vi "CreateMethod.vi"(0 "ClassWriterNative.lvclass":refnum<class "ClassWriterNative.lvclass">=refnum, 1 "ClassItemRefIn":refnum<vi>, 2 "CreateMethodData":T1={"MethodName"="", "RelativeMethodPath"=path "", "MethodDescription"="", "Scope/Visibility"=enum."Use Parent Folder Scope", "MethodTemplateName"="", "IconOut"=[], "RelativeProjectClassPath"="", "OpenViAfterCreation"=FALSE, "DynamicDispatchVi"=FALSE, "ExtraCreateParameters"=variant, "MustOverride"=FALSE, "MustCallParent"=FALSE, "IconDetails"={"IconSize"=enum."1 c-term high", "ImageRows(32)"=32, "ConnectorPaneHeight"=[]}, "AF-Option"=variant, "TemplatePath"=path ""} {"IconOut" format="%x"}, 5 "error in (no error)":errorcluster) -> (14 "ClassWriterNative.lvclass 2":refnum<class "ClassWriterNative.lvclass">, 15 "ClassItemRefOut":refnum<vi>, 16 "MethodPaths":path[](array[path]), 19 "error out":errorcluster)   [LabVIEW 2020, in "ClassWriterNative.lvclass"]
uses:
  ClassWriterNative.lvclass
  <vilib>/regexp/Match Regular Expression.xnode
  <vilib>/picture/picture.llb/imagedata.ctl
  <resource>/Framework/Providers/Open_GDS/ClassProviders/Common/LvIcon_class/GDSLvIcon_WordCompressionType.ctl
  <resource>/Framework/Providers/Open_GDS/ClassProviders/Common/LvIcon_class/subvis/GDSLvIcon_TextDataType.ctl
  <resource>/Framework/Providers/Open_GDS/ClassProviders/Provider_EndevoGOOP300/GOOP300_SubVIs/GOOP300_MethodScopeType.ctl
  <resource>/Framework/Providers/Open_GDS/ClassProviders/Provider_BaseClassInterface/BaseProvider_SubVIs/BaseProvider_PlugInManagerActions.ctl
  <vilib>/Utility/config.llb/NI_LVConfig.lvlib
  <resource>/Framework/Providers/Open_GDS/ClassProviders/Common/ScriptingFunctions/Scripting_ConnectorPanePatternType.ctl
  <vilib>/Utility/lvfile.llb/NI_FileType.lvlib
  <resource>/Framework/Providers/Open_GDS/ClassProviders/Common/LvClass_class/GDSLvClass_PlugInTypes.ctl
  <resource>/Framework/Providers/Open_GDS/ClassProviders/Common/LvClass_class/GDSLvClass_PlugIn.ctl
  <resource>/Framework/Providers/Open_GDS/ClassProviders/Provider_BaseClassInterface/BaseProvider_SubVIs/BaseProvider_DesignPatternsActions.ctl
  <resource>/Framework/Providers/Open_GDS/ClassProviders/Common/LvIcon_class/GDSLvIcon_TextAlignment.ctl
  <resource>/Framework/Providers/Open_GDS/ClassProviders/Provider_LvNativeClass/ClassWriterNative_class/MethodType.ctl
  <resource>/Framework/Providers/Open_GDS/ClassProviders/Provider_BaseClassInterface/ClassWriter_class/TemplateSettings.ctl
  Common/ScriptingFunctions/Scripting.lvclass
  <vilib>/Utility/config.llb/Read Key (String).vi
  <resource>/Framework/Providers/Open_GDS/ClassProviders/Provider_EndevoGOOP400/EndevoG4ProviderName.ctl
  <resource>/Framework/Providers/Open_GDS/ClassProviders/Provider_BaseClassInterface/CreateMethodData.ctl
  <resource>/Framework/Providers/Open_GDS/ClassProviders/Provider_LvNativeClass/ClassWriterNative_class/IconSize.ctl
  <resource>/Framework/Providers/Open_GDS/ClassProviders/Provider_LvNativeClass/ClassWriterNative_class/IconDetails.ctl
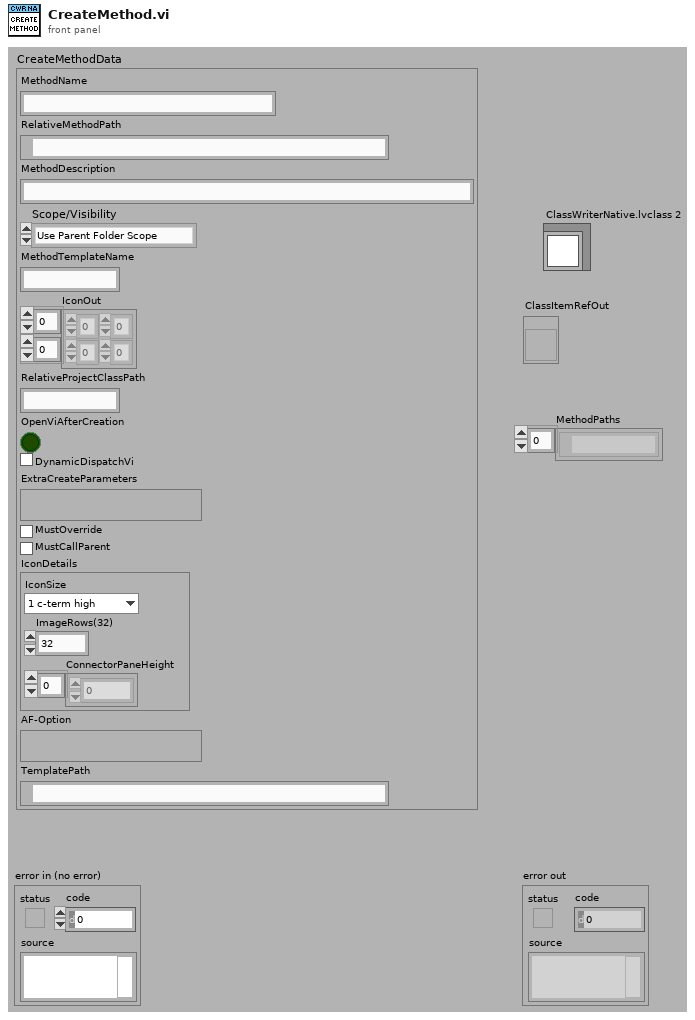
[diagram p1: front panel]
types:
  T1 = typedef "ClassWriter.lvclass/CreateMethodData.ctl" = cluster{"MethodName":string, "RelativeMethodPath":path, "MethodDescription":string, "Scope/Visibility":T2, "MethodTemplateName":string, "IconOut":u8[][], "RelativeProjectClassPath":string, "OpenViAfterCreation":bool, "DynamicDispatchVi":bool, "ExtraCreateParameters":variant, "MustOverride":bool, "MustCallParent":bool, "IconDetails":T3, "AF-Option":variant, "TemplatePath":path}
  T2 = typedef "GOOP300_MethodScopeType.ctl" = enum16{"Use Parent Folder Scope", "Public", "Protected", "Private", "Community"}
  T3 = typedef "ClassWriterNative.lvclass/IconDetails.ctl" = cluster{"IconSize":T4, "ImageRows(32)":i32, "ConnectorPaneHeight":i32[]}
  T4 = typedef "ClassWriterNative.lvclass/IconSize.ctl" = enum16{"Full", "1 c-term high", "2 c-term high", "3 c-term high"}
  T5 = typedef "ClassWriter.lvclass/TemplateSettings.ctl" = cluster{"CommonClassTemplate":bool, "DynamicDispatch":enum8{"False", "True", "Mixed"}, "MustOverride":enum8{"False", "True", "Mixed"}, "MustCallParent":enum8{"False", "True", "Mixed"}, "OnlyNormalMethod":bool, "OnlyPublic":bool}
  T6 = typedef "GDSLvClass_PlugIn.ctl" = cluster{"Type":T7, "ID":string, "Version":string, "Path":path, "Name":string, "Data":variant}
  T7 = typedef "GDSLvClass_PlugInTypes.ctl" = enum16{"DesignPattern", "MethodTypes"}
  T8 = cluster{"NewVIPath":path, "TemplateName":string, "VI":refnum<vi>, "ProjectFolder":refnum<vi>, "Library":refnum<vi>, "DestroyProjectFolderItem":bool, "ViProjectItem":refnum<vi>, "Property":string, "OverrideVi":path, "OverrideVIRef":refnum<vi>, "PlugInCall":cluster{"PlugInName":string, "MethodSelected":string}, "TemplateFolder":path, "D-Pattern":T6, "DesignPattern":bool, "Scope":enum32{"invalid scope", "public", "private", "protected", "community"}, "App":refnum<vi>, "SubVIs":refnum<vi>[], "MethodType":enum16{"Normal", "Override", "Property", "Af-Method"}, "Af-TemplatePath":path, "PropertyNode":bool, "PropertyFolderName":string, "TemplateSettings":T5}
  T9 = typedef "EndevoG4ProviderName.ctl" = enum16{"EndevoGOOP400"}
  T10 = cluster{"AttributeNames":string[], "PropertyNode":bool, "FolderNames":string[]}
  T11 = cluster{"PlugInName":string, "MethodSelected":string}
  T12 = enum16{"Normal", "Override", "Property", "Af-Method"}
  T13 = typedef "ClassWriterNative.lvclass/MethodType.ctl" = enum16{"Normal", "MethodPlugIn", "DesignPattern", "AF-Method"}
  T14 = cluster{"Type":T13, "Path":path, "OverrideVi":path}
  T15 = typedef "BaseProvider_PlugInManagerActions.ctl" = enum16{"GetPluginsMethods", "ExecutePlugIn"}
  T16 = enum32{"invalid scope", "public", "private", "protected", "community"}
  T17 = enum8{"Include the clone VI", "Include the original reentrant VI instead of the clone VI", "Include both the original reentrant VI and the clone VI"}
  T18 = enum8{"No dynamic dispatch VIs", "Include nearest implementation", "Include all overrides"}
  T19 = enum8{"Only include commented out diagrams if diagram already loaded", "Never include commented out diagrams", "Always include commented out diagrams"}
  T20 = enum32{"invalid scope", "public", "private", "protected"}
  T21 = enum16{"Share clones between instances", "Preallocate clone for each instance"}
  T22 = enum16{"Invalid Wire Rule", "Required", "Recommended", "Optional", "Dynamic Dispatch"}
  T23 = typedef "imagedata.ctl" = cluster{"image type":i32, "image depth":i32, "image":u8[], "mask":u8[], "colors":u32[], "Rectangle":cluster{"left":i16, "top":i16, "right":i16, "bottom":i16}}
  T24 = typedef "GDSLvIcon_TextDataType.ctl" = cluster{"Text":string, "Allow Only Capital Chars":bool, "Compression":T25, "Alignment":T26}
  T25 = typedef "GDSLvIcon_WordCompressionType.ctl" = enum16{"Auto", "On", "Off"}
  T26 = typedef "GDSLvIcon_TextAlignment.ctl" = enum16{"Center", "Left", "Right"}
  T27 = typedef "BaseProvider_DesignPatternsActions.ctl" = enum16{"AddPatternDialog", "GeneratePattern", "RemovePattern", "CreatePatternMethod", "UpdatePattern"}
  T28 = typedef "GOOP400_Options.ctl" = cluster{"FlatFolderStructure":bool, "CleanUpBDForPropertyMethods":bool}
  T29 = typedef "GDSLvCLass_ClassSettingsType.ctl" = cluster{"ClassProviderName":string, "ClassTemplateUsed":string, "ClassTemplateVersion":string, "ClassDescription":string, "PlugIns":T6[], "ConnectorPanePattern":string}
  T30 = enum32{"invalid scope", "public", "private", "protected", "community"}[]
  T31 = typedef "LVRectTypeDef.ctl" = cluster{"Left":i16, "Top":i16, "Right":i16, "Bottom":i16}
  T32 = typedef "GDSLvClass_IconSettingsType.ctl" = cluster{"Frame":u32, "Frame thickness":u8, "Header Background":u32, "Header Text":u32, "ColorPublic":u32, "ColorProtected":u32, "ColorPrivate":u32, "Body Text":u32, "ClassBodyIcon":string}
  T33 = typedef "Scripting_ConnectorPanePatternType.ctl" = u16
  T34 = cluster{"CtrlRef":refnum<vi>, "BeforeTerminalIndex":i32, "AfterTerminalIndex":i32}[]
  T35 = typedef "NI_LVConfig.lvlib/Config Data RefNum.ctl" = refnum<k1>
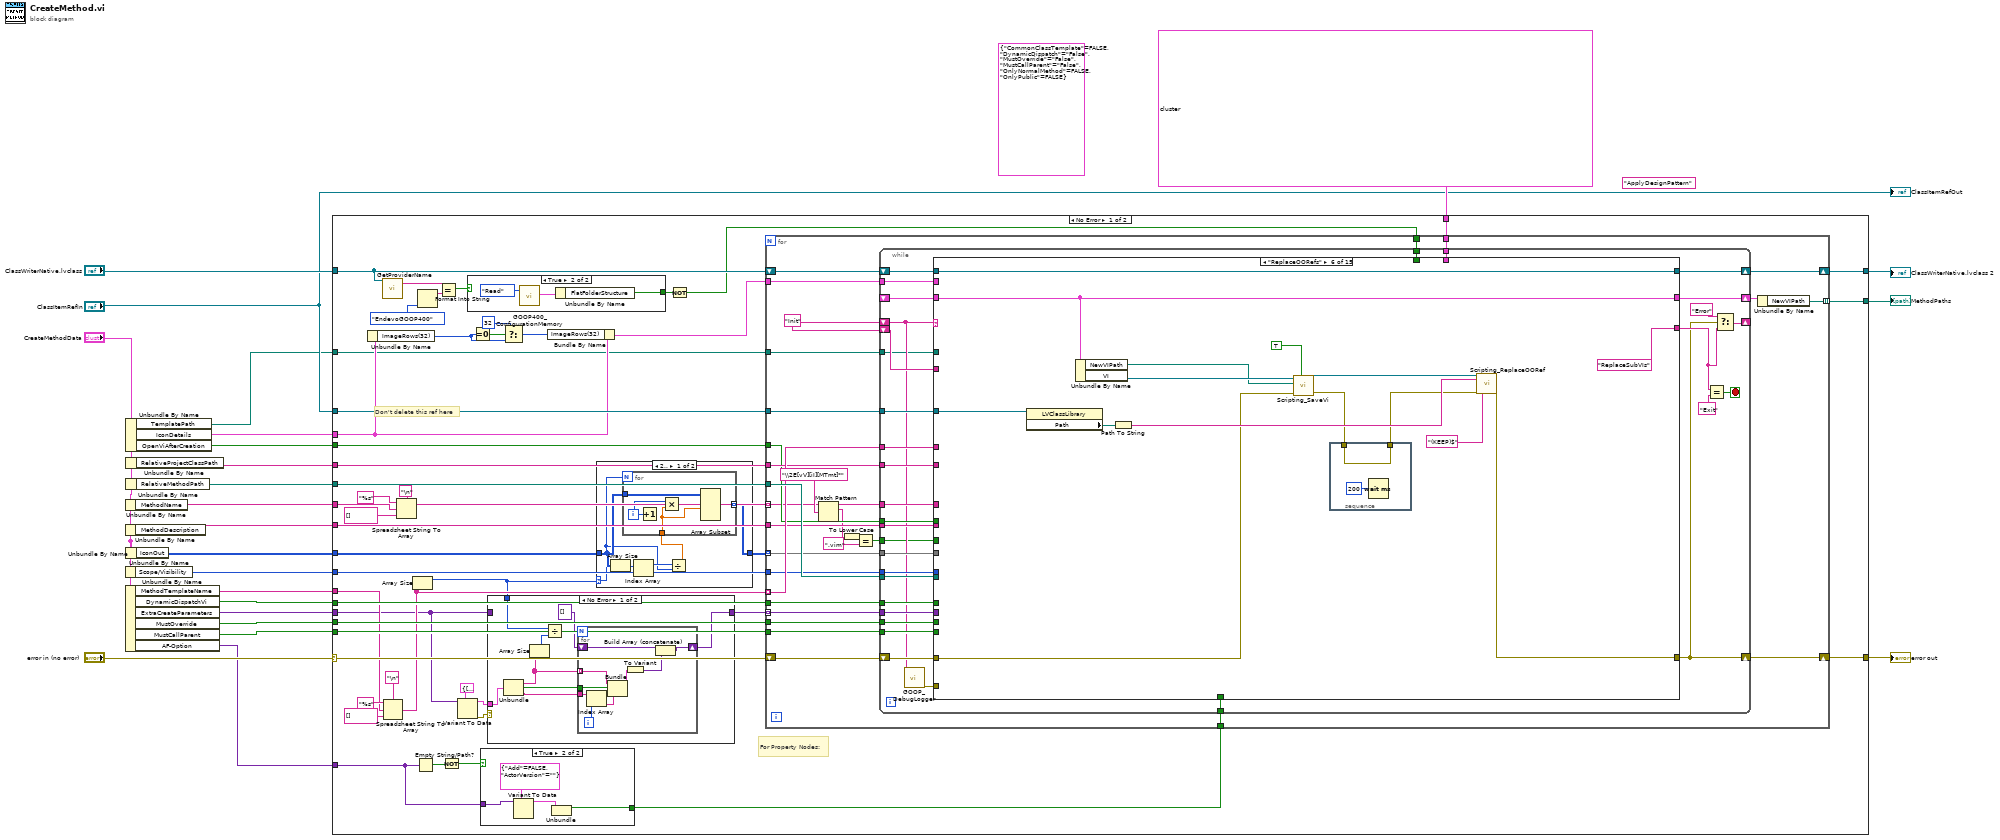
[diagram p0: block diagram]
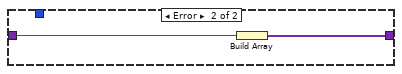
[diagram p4: hidden frame]
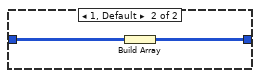
[diagram p5: hidden frame]
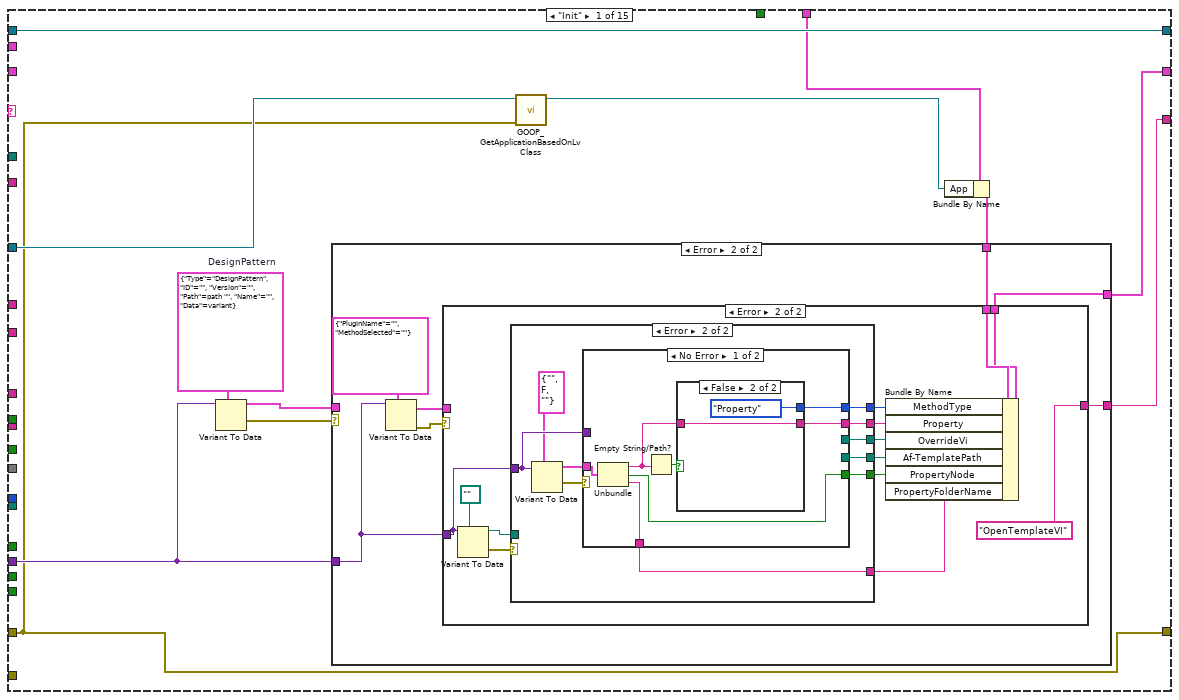
[diagram p6: hidden frame]
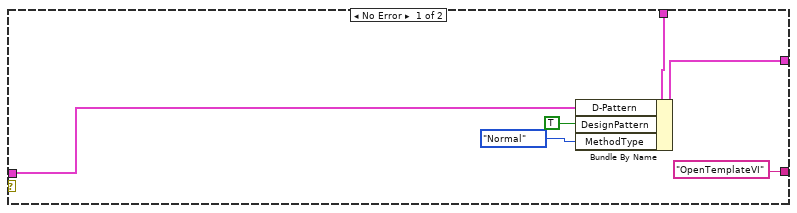
[diagram p7: hidden frame]
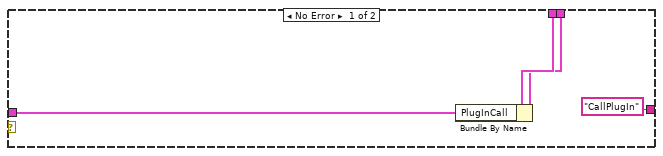
[diagram p8: hidden frame]
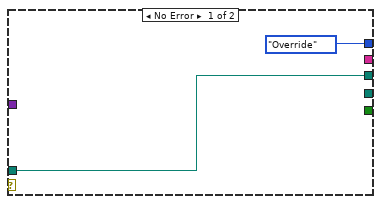
[diagram p9: hidden frame]
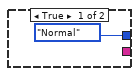
[diagram p10: hidden frame]
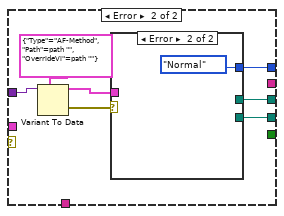
[diagram p11: hidden frame]
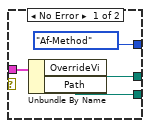
[diagram p12: hidden frame]
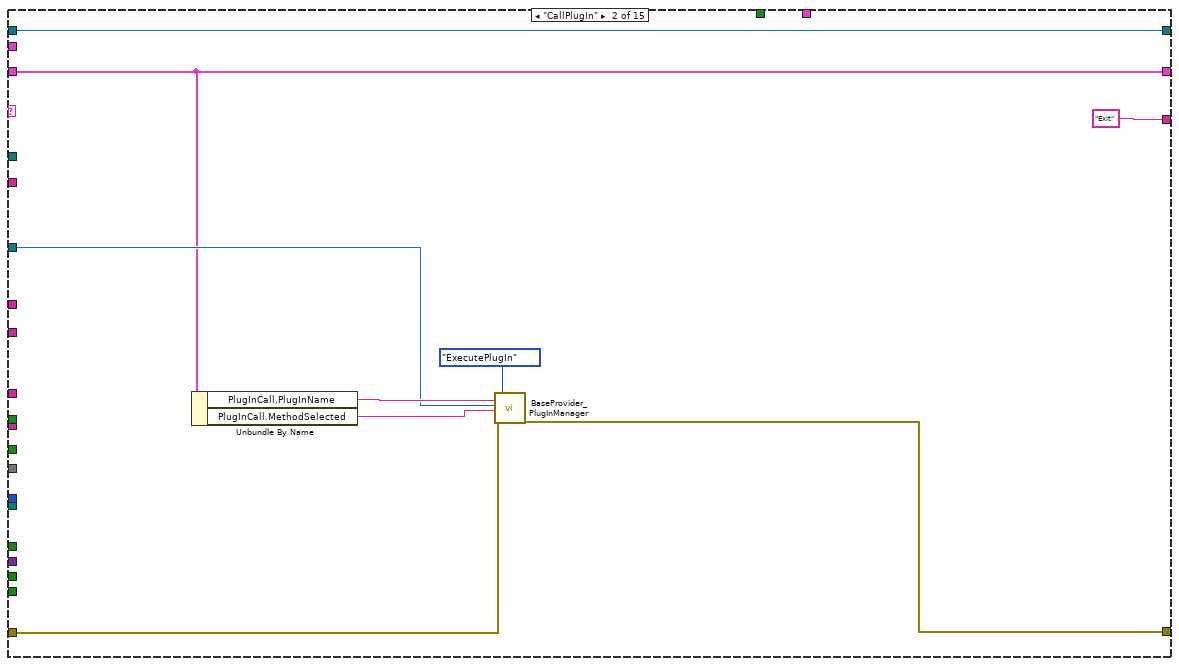
[diagram p13: hidden frame]
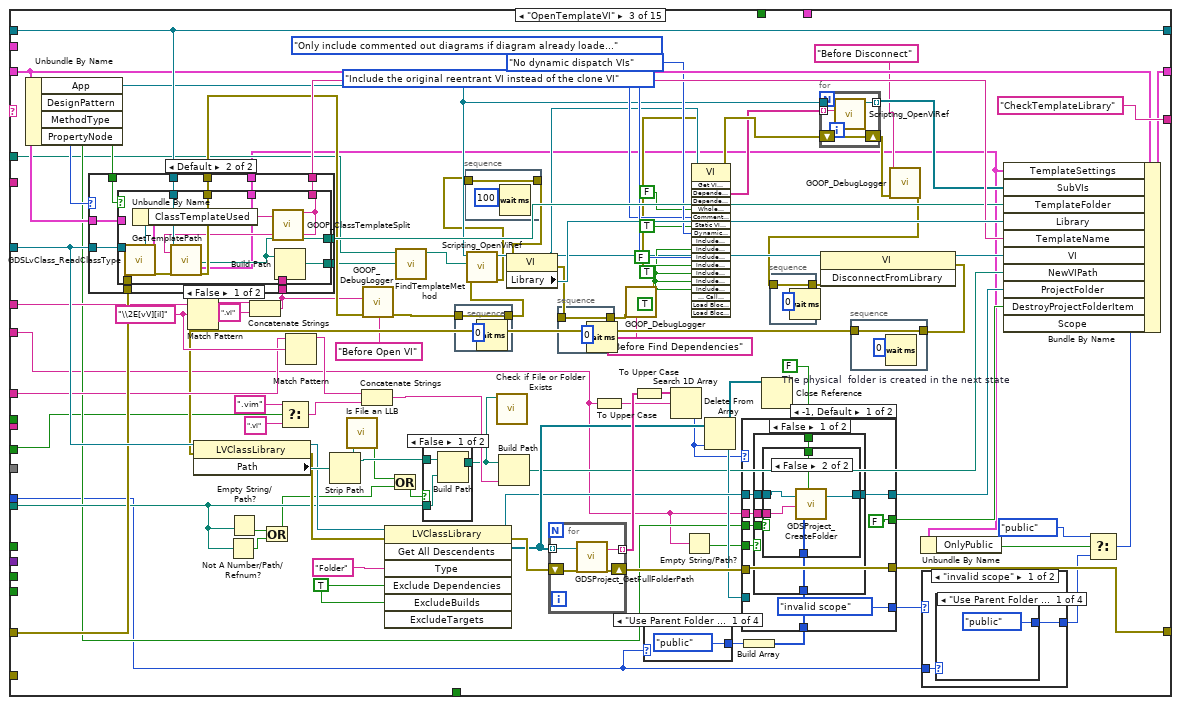
[diagram p14: hidden frame]
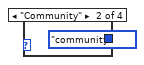
[diagram p15: hidden frame]
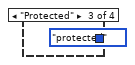
[diagram p16: hidden frame]
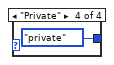
[diagram p17: hidden frame]
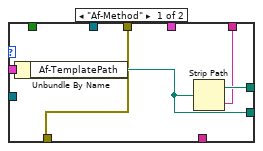
[diagram p18: hidden frame]
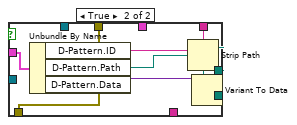
[diagram p19: hidden frame]
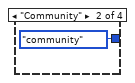
[diagram p20: hidden frame]
diagram:
  (unwired) T5 {"CommonClassTemplate"=FALSE, "DynamicDispatch"=enum."False", "MustOverride"=enum."False", "MustCallParent"=enum."False", "OnlyNormalMethod"=FALSE, "OnlyPublic"=FALSE} ("TemplateSettings")
  (unwired) "ApplyDesignPattern"
  n1 = Unbundle By Name("CreateMethodData") -> ("MethodName"=w14:string)
  n2 = Unbundle By Name("CreateMethodData") -> ("MethodDescription"=w15:string)
  n3 = Unbundle By Name("CreateMethodData") -> ("Scope/Visibility"=w11:T2)
  n4 = Unbundle By Name("CreateMethodData") -> ("MethodTemplateName"=w17:string, "DynamicDispatchVi"=w10:bool, "ExtraCreateParameters"=w9:variant, "MustOverride"=w6:bool, "MustCallParent"=w7:bool, "AF-Option"=w3:variant)
  n5 = Unbundle By Name("CreateMethodData") -> ("TemplatePath"=w2:path, "IconDetails"=w4:T3, "OpenViAfterCreation"=w18:bool)
  n6 = Unbundle By Name("CreateMethodData") -> ("RelativeProjectClassPath"=w12:string)
  n7 = Unbundle By Name("CreateMethodData") -> ("RelativeMethodPath"=w13:path)
  n8 = Unbundle By Name("CreateMethodData") -> ("IconOut"=w16:u8[][])
  n9 = case shown="No Error" "error in (no error)" {
    selector: "error in (no error)" -> [w73 w1229]
    tunnel: "ClassWriterNative.lvclass" -> [w30 w1228]
    tunnel: [w72 w1229] -> w22
    tunnel: [w70 w1228] -> w20
    tunnel: T8 {"NewVIPath"=path "", "TemplateName"="", "VI"=refnum, "ProjectFolder"=refnum, "Library"=refnum, "DestroyProjectFolderItem"=TRUE, "ViProjectItem"=refnum, "Property"="", "OverrideVi"=path "", "OverrideVIRef"=refnum, "PlugInCall"={"PlugInName"="", "MethodSelected"=""}, "TemplateFolder"=path "", "D-Pattern"={"Type"=enum."DesignPattern", "ID"="", "Version"="", "Path"=path "", "Name"="", "Data"=variant}, "DesignPattern"=FALSE, "Scope"=enum."invalid scope", "App"=refnum, "SubVIs"=[], "MethodType"=enum."Af-Method", "Af-TemplatePath"=path "", "PropertyNode"=FALSE, "PropertyFolderName"="", "TemplateSettings"={"CommonClassTemplate"=FALSE, "DynamicDispatch"=enum."False", "MustOverride"=enum."False", "MustCallParent"=enum."False", "OnlyNormalMethod"=FALSE, "OnlyPublic"=FALSE}} ("output cluster") -> [w71 _]
    tunnel: "ClassItemRefIn" -> [w69 _]
    tunnel: w14 -> [w52 _]
    tunnel: w13 -> [w68 _]
    tunnel: w17 -> [w57 _]
    tunnel: w16 -> [w50 _]
    tunnel: w11 -> [w67 _]
    tunnel: w12 -> [w66 _]
    tunnel: w15 -> [w65 _]
    tunnel: w18 -> [w64 _]
    tunnel: w10 -> [w63 _]
    tunnel: w9 -> [w46 _]
    tunnel: w7 -> [w62 _]
    tunnel: w6 -> [w61 _]
    tunnel: w4 -> [w36 _]
    tunnel: w3 -> [w43 _]
    tunnel: w2 -> [w32 _]
    tunnel: [w31 _] -> w1
    frame No Error {
      # "For Property Nodes:"
      # "Don't delete this ref here"
      n10 = Unbundle By Name(w36) -> ("ImageRows(32)"=w38:i32)
      n11 = call-dynamic "GetProviderName.vi"("ClassWriterNative in"=w30) -> ("ProviderName"=w28:string)  [unwired: 14 in, 4 out]
      n12 = Spreadsheet String To Array(delimiter (Tab)="\n", format string="%s", spreadsheet string=w57, array type (2D Dbl)=string[] []) -> (array=w51:string[])
      n13 = Spreadsheet String To Array(delimiter (Tab)="\n", format string="%s", spreadsheet string=w52, array type (2D Dbl)=string[] []) -> (array=w54:string[])
      n14 = Array Size(array=w51) -> (size(s)=w44:i32)
      n15 = Empty String/Path?(string/path=w43) -> (empty?=w42:bool)
      n16 = Format Into String(EndevoG4ProviderName."EndevoGOOP400" ("ProviderName")) -> (resulting string=w29:string)  [unwired: 3 in, 1 out]
      n17 = Equal?(x=w28, y=w29) -> (x = y?=w26:bool)
      n18 = Not(x=w42) -> (.not. x?=w41:bool)
      n19 = Variant To Data(type=T10 {"AttributeNames"=[], "PropertyNode"=FALSE, "FolderNames"=[]} ("cluster"), Variant=w46) -> (data=w47:T10, error out=w48:errorcluster)  [unwired: 1 in]
      n20 = case shown="True" w26 {
        tunnel: [_ w74] -> w25
        frame False {
        }
        frame True {
          n21 = call <resource>:"GOOP400_ConfigurationMemory.vi"("Action"=enum16{"Read", "Load", "Save"}."Read") -> ("OptionsOut"=w75:T28)  [unwired: 17 in, 1 out]
          n22 = Unbundle By Name(w75) -> ("FlatFolderStructure"=w74:bool)
        }
      }
      n23 = Equal To 0?(x=w38) -> (x = 0?=w39:bool)
      n24 = case shown="True" w41 {
        tunnel: w43 -> [_ w80]
        tunnel: [_ w77] -> w40
        frame False {
        }
        frame True {
          n25 = Variant To Data(type=cluster{"Add":bool, "ActorVersion":string} {"Add"=FALSE, "ActorVersion"=""} ("cluster"), Variant=w80) -> (data=w78:cluster{"Add":bool, "ActorVersion":string})  [unwired: 1 in, 1 out]
          n26 = Unbundle(w78) -> ("Add"=w77:bool)  [unwired: 1 out]
        }
      }
      n27 = case shown="No Error" w48 {
        tunnel: w47 -> [w84 _]
        tunnel: w46 -> [_ w99]
        tunnel: [w88 w98] -> w45
        tunnel: w44 -> [w86 _]
        frame No Error {
          n28 = Unbundle(w84) -> ("AttributeNames"=w83:string[], "PropertyNode"=w82:bool, "FolderNames"=w81:string[])
          n29 = Array Size(array=w83) -> (size(s)=w85:i32)
          n30 = Divide(x=w86, y=w85) -> ()  [unwired: 1 out]
          n31 = for {
            shift-right: [w96] -> w88
            shift-left: variant[] [] -> [w97]
            tunnel: w83 -> [w94] mode=indexing
            tunnel: w82 -> [w95]
            tunnel: w81 -> [w92]
            i -> [w91]
            n32 = Index Array(array=w92, index=w91) -> (element=w90:string)
            n33 = Bundle(w94, "PropertyNode"=w95, w90) -> (w93:cluster{string, "PropertyNode":bool, string})  [unwired: 1 in]
            n34 = To Variant(anything=w93) -> (Variant=w89:variant)
            n35 = Build Array (concatenate)(w97, w89) -> (w96:variant[])
          }
        }
        frame Error {
          n36 = Build Array(w99) -> (w98:variant[])
        }
      }
      n37 = Select(t=32, s=w39, f=w38) -> (s? t:f=w37:i32)
      n38 = Bundle By Name(cluster=w36, "ImageRows(32)"=w37) -> (w35:T3)
      n39 = case shown="2.." w44 {
        selector: w44 -> [w102 _]
        tunnel: w50 -> [w104 w112]
        tunnel: [w100 w111] -> w49
        frame 2.. {
          n40 = Array Size(array=w104) -> (size(s)=w105:i32[])
          n41 = Index Array(array=w105) -> (element=w103:i32)  [unwired: 1 in]
          n42 = Divide(x=w103, y=w102) -> (x/y=w101:dbl)
          n43 = for {
            N: w102 -> [_]
            tunnel: w104 -> [w109]
            tunnel: w101 -> [w107]
            tunnel: [w106] -> w100 mode=indexing
            i -> [w110]
            n44 = Increment(x=w110) -> ()  [unwired: 1 out]
            n45 = Multiply(x=w110, y=w107) -> (x*y=w108:dbl)
            n46 = Array Subset(array=w109, index (row)=w108, length (row)=w107) -> (w106:u8[][])  [unwired: 2 in]
          }
        }
        frame 1, Default {
          n47 = Build Array(w112) -> (w111:u8[][][])
        }
      }
      n48 = Not(x=w25) -> (.not. x?=w24:bool)
      n49 = for {
        tunnel: w71 -> [w141]
        tunnel: w69 -> [w138]
        tunnel: w68 -> [w137]
        tunnel: w51 -> [w136] mode=indexing
        tunnel: w54 -> [w118] mode=indexing
        tunnel: w49 -> [w135] mode=indexing
        tunnel: w67 -> [w134]
        tunnel: w66 -> [w133]
        tunnel: w65 -> [w132]
        tunnel: w64 -> [w131]
        tunnel: w63 -> [w130]
        tunnel: w45 -> [w129] mode=indexing
        tunnel: w62 -> [w127]
        tunnel: w61 -> [w126]
        shift-right: [w142] -> w72
        shift-left: w73 -> [w143]
        shift-right: [w139] -> w70
        shift-left: w30 -> [w140]
        tunnel: w35 -> [w125]
        tunnel: w40 -> [w124]
        tunnel: w32 -> [w123]
        tunnel: [w121] -> w31 mode=indexing
        tunnel: w24 -> [w113]
        w128 = "Init"
        n50 = Match Pattern(string=w118, regular expression="\\2E[vV][iI][MTmt]*") -> (before substring=w119:string, match substring=w117:string)  [unwired: 1 in, 2 out]
        n51 = To Lower Case(string=w117) -> (all lower case string=w116:string)
        n52 = Equal?(x=w116, y=".vim") -> (x = y?=w114:bool)
        n53 = while {
          shift-right: [w165] -> w142
          shift-left: w143 -> [w176]
          shift-right: [w171] -> _
          shift-left: w128 -> [w150]
          shift-right: [w174] -> w122
          shift-left: _ -> [w175]
          tunnel: w141 -> [w169]
          shift-right: [w167] -> w139
          shift-left: w140 -> [w166]
          tunnel: w138 -> [w164]
          tunnel: w136 -> [w163]
          tunnel: w137 -> [w162]
          tunnel: w119 -> [w161]
          tunnel: w135 -> [w160]
          tunnel: w134 -> [w159]
          tunnel: w133 -> [w158]
          tunnel: w132 -> [w157]
          tunnel: w131 -> [w156]
          tunnel: w130 -> [w155]
          tunnel: w129 -> [w154]
          shift-left: w128 -> [w153]
          tunnel: w127 -> [w152]
          tunnel: w126 -> [w151]
          tunnel: w125 -> [w148]
          tunnel: w124 -> [w147]
          tunnel: w123 -> [w146]
          tunnel: w114 -> [w145]
          tunnel: w113 -> [w144]
          stop <- w172 stop-if-true
          n54 = call <resource>:"GOOP_DebugLogger.vi"("State"=w150) -> ("error out"=w149:errorcluster)  [unwired: 8 in, 2 out]
          n55 = case shown="\"ReplaceOORefs\"" w150 {
            selector: w150 -> [_ _ _ _ _ _ _ _ _ _ _ _ _ _ w1185]
            tunnel: w175 -> [_ w253 w313 w464 w509 w603 w632 w685 w708 w819 w1006 w1027 w1066 w1089 w1182]
            tunnel: [w182 w253 w354 w463 w515 w603 w632 w686 w708 w819 w1006 w1027 w1066 w1089 w1182] -> w174
            tunnel: w176 -> [w178 w259 w348 w460 w511 w597 w611 w683 w728 w816 w1007 w1029 w1069 w1093 w1190]
            tunnel: [w178 w254 w318 w459 w508 w599 w623 w677 w709 w800 w1001 w1028 w1068 w1088 w1184] -> w165
            tunnel: [w187 "Exit" "CheckTemplateLibrary" "OverrideVi?" "ReplaceOORefs" "ReplaceSubVIs" "AddViToProject" "CheckDynamicDispatch" ("t") "UpdateIcon" ("t") "UpdateDescription" "ChangeConnectorPaneLayoutToMatchNewIconSize" ("t") w1033 "CloseRefs" "CloseRefs" "Exit"] -> w168
            tunnel: w169 -> [w177 _ _ _ _ _ _ _ _ _ _ _ _ _ _]
            tunnel: [w188 w260 w324 w462 w513 w604 w622 w690 w727 w818 w1005 w1036 w1065 w1085 w1195] -> w167
            tunnel: w166 -> [w188 w260 w324 w462 w513 w604 w622 w690 w727 w818 w1005 w1036 w1065 w1085 w1195]
            tunnel: w164 -> [w180 w255 w356 _ w510 w602 w631 w662 w729 w817 w1000 _ w1067 w1090 w1174]
            tunnel: w163 -> [_ _ w330 _ _ _ _ _ _ _ _ _ _ w1086 _]
            tunnel: w162 -> [_ _ w338 _ _ _ _ _ _ _ _ _ _ _ _]
            tunnel: w161 -> [_ _ w327 _ _ _ _ _ _ w782 _ _ _ _ _]
            tunnel: w160 -> [_ _ _ _ _ _ _ _ _ w807 _ _ _ _ _]
            tunnel: w159 -> [_ _ w277 _ _ _ _ _ _ w803 _ _ _ _ _]
            tunnel: w158 -> [_ _ w274 _ _ _ _ _ _ _ _ _ _ _ _]
            tunnel: w157 -> [_ _ _ _ _ _ _ _ _ _ w1008 _ _ _ _]
            tunnel: w156 -> [_ _ _ _ _ _ _ _ _ _ _ _ _ _ w1189]
            tunnel: w155 -> [_ _ _ _ _ _ _ _ w705 _ _ _ _ _ _]
            tunnel: w154 -> [w186 _ _ _ _ _ _ _ _ _ _ _ _ _ _]
            tunnel: w153 -> [_ _ _ _ _ _ _ _ _ _ _ _ _ _ w1183]
            tunnel: w152 -> [_ _ _ _ _ _ _ w671 _ _ _ _ _ _ _]
            tunnel: w151 -> [_ _ _ _ _ _ _ w672 _ _ _ _ _ _ _]
            tunnel: w149 -> [_ _ _ _ _ _ _ _ _ _ _ _ _ _ _]
            tunnel: w148 -> [_ _ _ _ _ _ _ _ _ w788 _ w1031 _ _ _]
            tunnel: w147 -> [_ _ _ _ _ _ _ _ _ _ _ _ _ _ w1176]
            tunnel: w146 -> [_ _ w278 _ _ _ _ _ _ _ _ _ _ _ _]
            tunnel: w145 -> [_ _ w267 _ _ _ _ _ w711 _ _ _ _ _ _]
            tunnel: w144 -> [_ _ _ _ w506 _ _ _ _ _ _ _ _ _ _]
            frame "Init" {
              w185 = T6 {"Type"=enum."DesignPattern", "ID"="", "Version"="", "Path"=path "", "Name"="", "Data"=variant}  # DesignPattern
              n56 = Variant To Data(type=w185, Variant=w186) -> (data=w183:T6, error out=w184:errorcluster)  [unwired: 1 in]
              n57 = call <resource>:"GOOP_GetApplicationBasedOnLvClass.vi"("error in (no error)"=w178, "LVClassLibrary in"=w180) -> ("Application out"=w179:refnum<vi>)  [unwired: 8 in, 1 out]
              n58 = Bundle By Name(cluster=w177, "App"=w179) -> (w181:T8)
              n59 = case shown="Error" w184 {
                tunnel: w181 -> [w194 w201]
                tunnel: [w192 w195] -> w182
                tunnel: ["OpenTemplateVI" w197] -> w187
                tunnel: w186 -> [_ w196]
                tunnel: w183 -> [w193 _]
                frame No Error {
                  n60 = Bundle By Name(cluster=w194, "D-Pattern"=w193, "DesignPattern"=TRUE, "MethodType"=enum16{"Normal", "Override", "Property"}."Normal") -> (w192:T8)
                }
                frame Error {
                  n61 = Variant To Data(type=T11 {"PlugInName"="", "MethodSelected"=""}, Variant=w196) -> (data=w198:T11, error out=w199:errorcluster)  [unwired: 1 in]
                  n62 = case shown="Error" w199 {
                    tunnel: w201 -> [w205 w218]
                    tunnel: [w204 w217] -> w195
                    tunnel: w196 -> [_ w209]
                    tunnel: w198 -> [w203 _]
                    tunnel: ["CallPlugIn" "OpenTemplateVI"] -> w197
                    frame No Error {
                      n63 = Bundle By Name(cluster=w205, "PlugInCall"=w203) -> (w204:T8)
                    }
                    frame Error {
                      n64 = Variant To Data(type=path "", Variant=w209) -> (data=w212:path, error out=w215:errorcluster)  [unwired: 1 in]
                      n65 = case shown="Error" w215 {
                        tunnel: [T12."Override" ("MethodType") w230] -> w214
                        tunnel: w209 -> [_ w226]
                        tunnel: [_ w229] -> w213
                        tunnel: w212 -> [w220 _]
                        tunnel: [w220 w225] -> w211
                        tunnel: [_ w224] -> w208
                        tunnel: [_ w222] -> w207
                        tunnel: [_ w221] -> w206
                        frame No Error {
                        }
                        frame Error {
                          n66 = Variant To Data(type=cluster{string, bool, string} {"", FALSE, ""} ("output cluster"), Variant=w226) -> (data=w227:cluster{string, bool, string}, error out=w228:errorcluster)  [unwired: 1 in]
                          n67 = case shown="No Error" w228 {
                            tunnel: [w237 w247] -> w230
                            tunnel: w227 -> [w234 _]
                            tunnel: [w235 _] -> w229
                            tunnel: w226 -> [_ w246]
                            tunnel: [_ w242] -> w225
                            tunnel: [_ w241] -> w224
                            tunnel: [w232 _] -> w222
                            tunnel: [w231 _] -> w221
                            frame No Error {
                              n68 = Unbundle(w234) -> (w233:string, w232:bool, w231:string)
                              n69 = Empty String/Path?(string/path=w233) -> (empty?=w236:bool)
                              n70 = case shown="False" w236 {
                                tunnel: [T12."Normal" ("MethodType") T12."Property" ("MethodType")] -> w237
                                tunnel: [_ w240] -> w235
                                tunnel: w233 -> [_ w240]
                                frame True {
                                }
                                frame False {
                                }
                              }
                            }
                            frame Error {
                              n71 = Variant To Data(type=T14 {"Type"=enum."AF-Method", "Path"=path "", "OverrideVi"=path ""} ("output cluster"), Variant=w246) -> (data=w243:T14, error out=w244:errorcluster)  [unwired: 1 in]
                              n72 = case shown="Error" w244 {
                                tunnel: [T12."Af-Method" ("MethodType") T12."Normal" ("MethodType")] -> w247
                                tunnel: w243 -> [w250 _]
                                tunnel: [w249 _] -> w242
                                tunnel: [w248 _] -> w241
                                frame No Error {
                                n73 = Unbundle By Name(w250) -> ("OverrideVi"=w249:path, "Path"=w248:path)
                                }
                                frame Error {
                                }
                              }
                            }
                          }
                        }
                      }
                      n74 = Bundle By Name(cluster=w218, "MethodType"=w214, "Property"=w213, "OverrideVi"=w211, "Af-TemplatePath"=w208, "PropertyNode"=w207, "PropertyFolderName"=w206) -> (w217:T8)
                    }
                  }
                }
              }
            }
            frame "CallPlugIn" {
              n75 = Unbundle By Name(w253) -> ("PlugInCall.PlugInName"=w257:string, "PlugInCall.MethodSelected"=w256:string)
              n76 = call <resource>:"BaseProvider_PlugInManager.vi"("PlugInName"=w257, "ClassRefToActOn"=w255, "ExtraExInfo"=w256, "error in (no error)"=w259, "Action"=BaseProvider_PlugInManagerActions."ExecutePlugIn") -> ("error out"=w254:errorcluster)  [unwired: 13 in, 1 out]
            }
            frame "OpenTemplateVI" {
              w262 = FALSE  # The physical  folder is created in the next state
              w311 = TRUE ("Include Poly VIs?")
              w323 = TRUE ("ExcludeDependencies")
              w328 = "\\2E[vV][iI]" ("regular expression")
              n77 = Unbundle By Name(w313) -> ("App"=w300:refnum<vi>, "DesignPattern"=w314:bool, "MethodType"=w282:T12, "PropertyNode"=w281:bool)
              n78 = Match Pattern(string=w330, regular expression=w328) -> (before substring=w329:string)  [unwired: 1 in, 3 out]
              n79 = Not A Number/Path/Refnum?(number/path/refnum=w338) -> (NaN/Path/Refnum?=w336:bool)
              n80 = Empty String/Path?(string/path=w338) -> (empty?=w337:bool)
              n81 = Concatenate Strings(w329, ".vi" ("string")) -> (w291:string)
              n82 = case shown="Default" w282 {
                tunnel: w356 -> [_ w378]
                tunnel: w348 -> [w364 w377]
                tunnel: [w363 w376] -> w331
                tunnel: w324 -> [_ w375]
                tunnel: [w366 w374] -> w280
                tunnel: [w365 w373] -> w315
                tunnel: w314 -> [_ w372]
                tunnel: w313 -> [w367 w371]
                tunnel: [w364 w370] -> w293
                tunnel: w291 -> [_ w369]
                tunnel: [_ w368] -> w272
                frame "Af-Method" {
                  n83 = Unbundle By Name(w367) -> ("Af-TemplatePath"=w366:path)
                  n84 = Strip Path(path=w366) -> (stripped path=w365:path, name=w363:string)
                }
                frame Default {
                  n85 = case shown="False" w372 {
                    tunnel: [w389 w397] -> w370
                    tunnel: w378 -> [w380 _]
                    tunnel: w369 -> [w388 _]
                    tunnel: w377 -> [w387 w397]
                    tunnel: [w381 w395] -> w376
                    tunnel: w375 -> [w385 _]
                    tunnel: [w384 w391] -> w374
                    tunnel: [w383 w394] -> w373
                    tunnel: w371 -> [_ w396]
                    tunnel: [w379 _] -> w368
                    frame False {
                      n86 = call <resource>:"GDSLvClass_ReadClassType.vi"("Class Refnum In"=w380, "error in (no error)"=w387) -> ("ClassSettings"=w386:T29, "error out"=w390:errorcluster)  [unwired: 15 in, 1 out]
                      n87 = Unbundle By Name(w386) -> ("ClassTemplateUsed"=w382:string)
                      n88 = call <resource>:"GOOP_ClassTemplateSplit.vi"("ClassItemRefIn"=w380, "FullClassTemplate"=w382) -> ("StandardTemplate"=w381:string)  [unwired: 12 in, 1 out]
                      n89 = call-dynamic "GetTemplatePath.vi"("reference in"=w385, "ClassTemplateSubDirectory"=w381, "error in (no error)"=w390) -> ("MethodTemplatePathOut"=w383:path, "TemplateSettings"=w379:T5, "error out"=w389:errorcluster)  [unwired: 12 in, 2 out]
                      n90 = Build Path(base path=w383, name or relative path=w388) -> (appended path=w384:path)
                    }
                    frame True {
                      n91 = Unbundle By Name(w396) -> ("D-Pattern.ID"=w395:string, "D-Pattern.Path"=w392:path, "D-Pattern.Data"=w393:variant)
                      n92 = Strip Path(path=w392) -> (stripped path=w394:path)  [unwired: 1 out]
                      n93 = Variant To Data(type=w392, Variant=w393) -> (data=w391:path)  [unwired: 1 in, 1 out]
                    }
                  }
                }
              }
              n94 = Or(x=w337, y=w336) -> (x .or. y?=w321:bool)
              n95 = Select(t=".vim" ("string"), s=w267, f=".vi" ("string")) -> (s? t:f=w264:string)
              n96 = Match Pattern(string=w327, regular expression=w328) -> (before substring=w326:string)  [unwired: 1 in, 3 out]
              n97 = Concatenate Strings(w326, w264) -> (w353:string)
              n98 = call <resource>:"GOOP_DebugLogger.vi"("error in (no error)"=w293, "Data"=w291, "State"="Before Open VI") -> ("error out"=w290:errorcluster)  [unwired: 6 in, 2 out]
              n99 = call <resource>:"FindTemplateMethod.vi"("TemplatePath To Use first"=w280, "TemplatePath in"=w278) -> ("TemplatePath out"=w279:path)  [unwired: 9 in]
              n100 = stacked-sequence {
                tunnel: w290 -> [w400]
                tunnel: [w400] -> w289
                frame #0 {
                  n101 = Wait (ms)(milliseconds to wait=u32 0) -> ()  [unwired: 1 out]
                }
              }
              n102 = call "Scripting_OpenViRef.vi"("error in"=w289, "ViPath/ViName/Viref"=w279, "AppRef"=w300) -> ("error out"=w284:errorcluster, "vi reference"=w312:refnum<vi>)  [unwired: 6 in, 1 out]
              n103 = stacked-sequence {
                tunnel: w284 -> [w398]
                tunnel: [w398] -> w283
                frame #0 {
                  n104 = Wait (ms)(milliseconds to wait=u32 100) -> ()  [unwired: 1 out]
                }
              }
              n105 = property class="VI"(reference=w312, error in=w283) -> (reference out=w303:refnum<vi>, error out=w288:errorcluster, "Library"=w340:refnum<vi>)
              n106 = stacked-sequence {
                tunnel: w288 -> [w402]
                tunnel: [w402] -> w286
                frame #0 {
                  n107 = Wait (ms)(milliseconds to wait=u32 0) -> ()  [unwired: 1 out]
                }
              }
              n108 = To Upper Case(1:w274) -> (0:w345:string)
              n109 = call <resource>:"GOOP_DebugLogger.vi"("error in (no error)"=w286, "State"="Before Find Dependencies") -> ("error out"=w285:errorcluster)  [unwired: 7 in, 2 out]
              n110 = case shown="\"Use Parent Folder Scope\", \"Public\"" w277 {
                tunnel: [T16."public" ("Source Scope:Get") T16."community" ("Source Scope:Get") T16."protected" ("Source Scope:Get") T16."private" ("Source Scope:Get")] -> w276
                frame "Use Parent Folder Scope", "Public" {
                }
                frame "Community" {
                }
                frame "Protected" {
                }
                frame "Private" {
                }
              }
              n111 = Empty String/Path?(string/path=w274) -> (empty?=w273:bool)
              n112 = invoke class="VI" method="Get VI Dependencies"(reference=w303, error in=w285, "Whole Hierarchy?"=FALSE, "Commented Out?"=T19."Only include commented out diagrams if diagram already loaded" ("Commented Out Diagrams?"), "Static VI Refs?"=TRUE, "Dynamic Dispatching?"=T18."No dynamic dispatch VIs", "Include Missing VIs?"=FALSE ("Include Missing Items?"), "Include Standard VIs?"=TRUE, "Include Reentrant Clones?"=T17."Include the original reentrant VI instead of the clone VI", "Include Poly VIs?"=w311, "Include Global VIs?"=w311, "Include Control VIs?"=w311, "Include Generic VIs?"=w311) -> (error out=w302:errorcluster, "Dependency Names"=w301:string[])  [unwired: 6 in, 17 out]
              n113 = Build Array(w276) -> (w275:T30)
              n114 = for {
                shift-right: [w409] -> w296
                shift-left: w302 -> [w409]
                tunnel: w301 -> [w408] mode=indexing
                tunnel: w300 -> [w407]
                tunnel: [w406] -> w299 mode=indexing
                n115 = call "Scripting_OpenViRef.vi"("ViPath/ViName/Viref"=w408, "AppRef"=w407) -> ("vi reference"=w406:refnum<vi>)  [unwired: 7 in, 2 out]
              }
              n116 = call <resource>:"GOOP_DebugLogger.vi"("error in (no error)"=w296, "State"="Before Disconnect") -> ("error out"=w295:errorcluster)  [unwired: 7 in, 2 out]
              n117 = stacked-sequence {
                tunnel: w295 -> [w410]
                tunnel: [w410] -> w317
                frame #0 {
                  n118 = Wait (ms)(milliseconds to wait=u32 0) -> ()  [unwired: 1 out]
                }
              }
              n119 = invoke class="VI" method="DisconnectFromLibrary"(reference=w303, error in=w317) -> (reference out=w332:refnum<vi>, error out=w298:errorcluster)  [unwired: 1 in, 1 out]
              n120 = stacked-sequence {
                tunnel: [w404] -> w297
                tunnel: w298 -> [w404]
                frame #0 {
                  n121 = Wait (ms)(milliseconds to wait=u32 0) -> ()  [unwired: 1 out]
                }
              }
              n122 = property class="LVClassLibrary"(reference=w356, error in=w297) -> (reference out=w351:refnum<vi>, error out=w349:errorcluster, "Path"=w355:path)
              n123 = Strip Path(path=w355) -> (stripped path=w322:path)  [unwired: 1 out]
              n124 = call <vilib>:"Is File an LLB.vi"("path"=w322) -> ("Is LLB?"=w320:bool)  [unwired: 9 in, 1 out]
              n125 = invoke class="LVClassLibrary" method="Get All Descendents"(reference=w351, error in=w349, "Type"="Folder", "Exclude Dependencies"=w323, "ExcludeBuilds"=w323) -> (reference out=w342:refnum<vi>, error out=w350:errorcluster, "All Descendents"=w344:refnum<vi>[])  [unwired: 2 in, 4 out]
              n126 = Or(x=w320, y=w321) -> (x .or. y?=w319:bool)
              n127 = case shown="False" w319 {
                tunnel: w322 -> [w453 w454]
                tunnel: [w452 w454] -> w263
                tunnel: w338 -> [w451 _]
                frame False {
                  n128 = Build Path(base path=w453, name or relative path=w451) -> (appended path=w452:path)
                }
                frame True {
                }
              }
              n129 = call <vilib>:"Check if File or Folder Exists.vi"("path"=w263) -> ()  [unwired: 8 in, 3 out]
              n130 = Build Path(base path=w263, name or relative path=w353) -> (appended path=w339:path)
              n131 = for {
                tunnel: w344 -> [w458] mode=indexing
                shift-right: [w456] -> w343
                shift-left: w350 -> [w457]
                tunnel: [w455] -> w347 mode=indexing
                n132 = call <resource>:"GDSProject_GetFullFolderPath.vi"("Folder Item"=w458, "error in (no error)"=w457) -> ("ProjectClassPath"=w455:string, "error out"=w456:errorcluster)  [unwired: 16 in]
              }
              n133 = To Upper Case(1:w347) -> (0:w346:string[])
              n134 = Search 1D Array(1D array=w346, element=w345) -> (index of element=w335:i32)  [unwired: 1 in]
              n135 = Delete From Array(array=w344, index=w335) -> (deleted portion=w341:refnum<vi>, array with subset deleted=w316:refnum<vi>[])  [unwired: 1 in]
              n136 = case shown="-1, Default" w335 {
                tunnel: w343 -> [w428 w450]
                tunnel: w342 -> [w424 w447]
                tunnel: w341 -> [_ w446]
                tunnel: [T16."invalid scope" ("Source Scope:Get") w449] -> w325
                tunnel: [w428 w448] -> w318
                tunnel: [w423 w446] -> w334
                tunnel: [FALSE TRUE] -> w333
                tunnel: w281 -> [w425 _]
                tunnel: w274 -> [w422 _]
                tunnel: w275 -> [w421 _]
                tunnel: w273 -> [w420 _]
                tunnel: w262 -> [w419 _]
                frame -1, Default {
                  n137 = case shown="False" w420 {
                    tunnel: w425 -> [w434 _]
                    tunnel: w424 -> [w433 w444]
                    tunnel: [w432 w444] -> w423
                    tunnel: w422 -> [w431 _]
                    tunnel: w421 -> [w430 _]
                    tunnel: w419 -> [w429 _]
                    frame False {
                      n138 = case shown="False" w434 {
                        tunnel: w433 -> [w438 w443]
                        tunnel: [w436 w441] -> w432
                        tunnel: w431 -> [w437 w442]
                        tunnel: w430 -> [_ w440]
                        tunnel: w429 -> [w435 w439]
                        frame True {
                          n139 = call <resource>:"GDSProject_CreateFolder.vi"("Project Item To Create Folder Below(Use MyComputer if not wired)"=w438, "FolderName"=w437, "CreateThePhysicalFolderIfPossible(False)"=w435) -> ("ItemOut"=w436:refnum<vi>)  [unwired: 13 in, 3 out]
                        }
                        frame False {
                          n140 = call <resource>:"GDSProject_CreateFolder.vi"("Project Item To Create Folder Below(Use MyComputer if not wired)"=w443, "FolderName"=w442, "FolderScope"=w440, "CreateThePhysicalFolderIfPossible(False)"=w439) -> ("ItemOut"=w441:refnum<vi>)  [unwired: 12 in, 3 out]
                        }
                      }
                    }
                    frame True {
                    }
                  }
                }
                frame 0.. {
                  n141 = invoke class="LVClassLibrary" method="Get Source Scope"(reference=w447, error in=w450, "SourceRef"=w446) -> (error out=w448:errorcluster, "GetSourceScope"=w449:T16)  [unwired: 2 in, 3 out]
                }
              }
              n142 = Close Reference(reference=w316) -> ()  [unwired: 1 in, 1 out]
              n143 = Unbundle By Name(w272) -> ("OnlyPublic"=w271:bool)
              n144 = case shown="\"invalid scope\"" w325 {
                selector: w325 -> [_ w418]
                tunnel: [w412 w418] -> w269
                tunnel: w277 -> [w413 _]
                frame "invalid scope" {
                  n145 = case shown="\"Use Parent Folder Scope\", \"Public\"" w413 {
                    tunnel: [T16."public" ("Source Scope:Get") T16."community" ("Source Scope:Get") T16."protected" ("Source Scope:Get") T16."private" ("Source Scope:Get")] -> w412
                    frame "Use Parent Folder Scope", "Public" {
                    }
                    frame "Community" {
                    }
                    frame "Protected" {
                    }
                    frame "Private" {
                    }
                  }
                }
                frame Default {
                }
              }
              n146 = Select(t=T16."public" ("Source Scope:Get"), s=w271, f=w269) -> (s? t:f=w270:T16)
              n147 = Bundle By Name(cluster=w313, "TemplateSettings"=w272, "SubVIs"=w299, "TemplateFolder"=w315, "Library"=w340, "TemplateName"=w331, "VI"=w332, "NewVIPath"=w339, "ProjectFolder"=w334, "DestroyProjectFolderItem"=w333, "Scope"=w270) -> (w354:T8)
            }
            frame "CheckTemplateLibrary" {
              n148 = Unbundle By Name(w464) -> ("Library"=w466:refnum<vi>, "TemplateFolder"=w461:path)
              n149 = Not A Number/Path/Refnum?(number/path/refnum=w466) -> (NaN/Path/Refnum?=w465:bool)
              n150 = case shown="True" w465 {
                tunnel: w464 -> [w469 w483]
                tunnel: [w469 w482] -> w463
                tunnel: w461 -> [_ w476]
                tunnel: w460 -> [w468 w471]
                tunnel: [w468 w470] -> w459
                frame False {
                }
                frame True {
                  n151 = Strip Path(path=w476) -> (stripped path=w475:path)  [unwired: 1 out]
                  n152 = List Folder(path=w476, pattern="*.lvclass") -> (path out=w479:path, filenames=w478:string[])  [unwired: 2 in, 2 out]
                  n153 = Array Size(array=w478) -> (size(s)=w480:i32)
                  n154 = Index Array(array=w478) -> (element=w477:string)  [unwired: 1 in]
                  n155 = case shown="1" w480 {
                    tunnel: w479 -> [_ w505]
                    tunnel: w477 -> [_ w504]
                    tunnel: w475 -> [w490 _]
                    tunnel: [w486 w502] -> w474
                    tunnel: w471 -> [w485 w501]
                    tunnel: [w484 w500] -> w470
                    frame 0, Default {
                      n156 = List Folder(path=w490, pattern="*.lvclass") -> (path out=w488:path, filenames=w492:string[])  [unwired: 2 in, 2 out]
                      n157 = Array Size(array=w492) -> (size(s)=w489:i32)
                      n158 = Index Array(array=w492) -> (element=w487:string)  [unwired: 1 in]
                      n159 = case shown="1" w489 {
                        tunnel: w488 -> [_ w498]
                        tunnel: w487 -> [_ w497]
                        tunnel: [_ w496] -> w486
                        tunnel: w485 -> [w493 w495]
                        tunnel: [w493 w494] -> w484
                        frame 0, Default {
                        }
                        frame 1 {
                          n160 = Build Path(base path=w498, name or relative path=w497) -> (appended path=w499:path)
                          n161 = call <resource>:"GDSLvClass_OpenClass.vi"("ClassToOpen"=w499, "error in (no error)"=w495) -> ("LVClass.Open"=w496:refnum<vi>, "error out"=w494:errorcluster)  [unwired: 16 in]
                        }
                      }
                    }
                    frame 1 {
                      n162 = Build Path(base path=w505, name or relative path=w504) -> (appended path=w503:path)
                      n163 = call <resource>:"GDSLvClass_OpenClass.vi"("ClassToOpen"=w503, "error in (no error)"=w501) -> ("LVClass.Open"=w502:refnum<vi>, "error out"=w500:errorcluster)  [unwired: 16 in]
                    }
                  }
                  n164 = To More Generic Class(target class=refnum<vi> refnum ("Library"), reference=w474) -> (generic class reference=w473:refnum<vi>)
                  n165 = Bundle By Name(cluster=w483, "Library"=w473) -> (w482:T8)
                }
              }
            }
            frame "OverrideVi?" {
              n166 = Unbundle By Name(w509) -> ("App"=w507:refnum<vi>, "OverrideVi"=w512:path)
              n167 = Empty String/Path?(string/path=w512) -> (empty?=w514:bool)
              n168 = case shown="False" w514 {
                tunnel: w509 -> [w558 w590]
                tunnel: [w557 w590] -> w515
                tunnel: w512 -> [w543 _]
                tunnel: w511 -> [w556 w589]
                tunnel: w510 -> [w531 _]
                tunnel: w509 -> [_ _]
                tunnel: [w522 w589] -> w508
                tunnel: w507 -> [w523 _]
                tunnel: w506 -> [w517 _]
                frame False {
                  n169 = call "Scripting_OpenViRef.vi"("error in"=w556, "ViPath/ViName/Viref"=w543, "AppRef"=w523) -> ("error out"=w549:errorcluster, "vi reference"=w547:refnum<vi>)  [unwired: 6 in, 1 out]
                  n170 = property class="VI"(reference=w547, error in=w549) -> (error out=w554:errorcluster, "Library"=w526:refnum<vi>)  [unwired: 1 out]
                  n171 = property class="Library"(reference=w526, error in=w554) -> (error out=w555:errorcluster, "Path"=w553:path)  [unwired: 1 out]
                  n172 = property class="VI"(reference=w547, error in=w555) -> (error out=w548:errorcluster, "Path"=w552:path)  [unwired: 1 out]
                  n173 = property class="LVClassLibrary"(reference=w531, error in=w548) -> (error out=w545:errorcluster, "Path"=w551:path)  [unwired: 1 out]
                  n174 = invoke class="Library" method="Get All Descendents"(reference=w526, error in=w545, "Type"="VI") -> (reference out=w541:refnum<vi>, error out=w524:errorcluster, "All Descendents"=w540:refnum<vi>[])  [unwired: 4 in, 4 out]
                  n175 = for {
                    tunnel: w540 -> [w588] mode=indexing
                    tunnel: [w587] -> w544 mode=indexing
                    n176 = property class="ProjectItem"(reference=w588) -> ("Path"=w587:path)  [unwired: 1 in, 2 out]
                  }
                  n177 = Search 1D Array(1D array=w544, element=w543) -> (index of element=w542:i32)  [unwired: 1 in]
                  n178 = Index Array(array=w540, index=w542) -> (element=w530:refnum<vi>)
                  n179 = while {
                    tunnel: [w578] -> w539 mode=indexing
                    shift-right: [w580] -> _
                    shift-left: w530 -> [w584]
                    tunnel: w526 -> [w583]
                    tunnel: [w581] -> w528 mode=indexing
                    tunnel: [w580] -> w525 mode=indexing
                    tunnel: [w576] -> w520
                    stop <- w585 continue-if-true
                    n180 = property class="ProjectItem"(reference=w584) -> ("Parent"=w582:refnum<vi>)  [unwired: 1 in, 2 out]
                    n181 = property class="ProjectItem"(reference=w582) -> (reference out=w580:refnum<vi>, "Name"=w578:string, "Type String"=w579:string)  [unwired: 1 in, 1 out]
                    n182 = Equal?(x=w579, y="Property Definition" ("Type")) -> (x = y?=w576:bool)
                    n183 = Equal?(x=w579, y="Folder") -> (x = y?=w585:bool)
                    n184 = invoke class="Library" method="Get Source Scope"(reference=w583, "SourceRef"=w582) -> ("GetSourceScope"=w581:T16)  [unwired: 3 in, 4 out]
                  }
                  n185 = invoke class="Library" method="Get Source Scope"(reference=w526, "SourceRef"=w530) -> ("GetSourceScope"=w529:T16)  [unwired: 3 in, 4 out]
                  n186 = call <vilib>:"Compare Two Paths.vi"("Path 2"=w552, "Path 1"=w553) -> ("Relative Path from 1 to 2"=w550:path)  [unwired: 6 in, 3 out]
                  n187 = case shown="True" w520 {
                    tunnel: w539 -> [w565 w573]
                    tunnel: [w563 "properties" ("trimmed string")] -> w534
                    tunnel: w528 -> [w561 w572]
                    tunnel: [w559 w572] -> w527
                    tunnel: [_ w571] -> w519
                    tunnel: [_ TRUE ("CreateThePhysicalFolderIfPossible(False)")] -> w518
                    frame False {
                      n188 = Delete From Array(array=w565) -> (array with subset deleted=w564:string[])  [unwired: 2 in, 1 out]
                      n189 = Delete From Array(array=w561) -> (array with subset deleted=w560:T30)  [unwired: 2 in, 1 out]
                      n190 = Reverse 1D Array(array=w564) -> (reversed array=w562:string[])
                      n191 = Reverse 1D Array(array=w560) -> (reversed array=w559:T30)
                      n192 = Array To Spreadsheet String(delimiter (Tab)="/", array=w562, 3:"%s" ("format string")) -> (spreadsheet string=w566:string)
                      n193 = call <vilib>:"Trim Whitespace.vi"("string"=w566) -> ("trimmed string"=w563:string)  [unwired: 1 in]
                    }
                    frame True {
                      n194 = Index Array(array=w573) -> (element=w571:string)  [unwired: 1 in]
                    }
                  }
                  n195 = Build Array (concatenate)(w540, w525) -> (w521:refnum<vi>[])
                  n196 = Build Path(base path=w551, name or relative path=w550) -> (appended path=w538:path)
                  n197 = Empty String/Path?(string/path=w534) -> (empty?=w536:bool)
                  n198 = call <resource>:"GDSProject_CreateFolder.vi"("Project Item To Create Folder Below(Use MyComputer if not wired)"=w531, "FolderName"=w534, "error in (no error)"=w524, "FolderScope"=w527, "CreateThePhysicalFolderIfPossible(False)"=w517) -> ("ItemOut"=w537:refnum<vi>, "error out"=w522:errorcluster)  [unwired: 11 in, 2 out]
                  n199 = invoke class="LVClassLibrary" method="Get Source Scope"(reference=w531, "SourceRef"=w537) -> ("GetSourceScope"=w533:T16)  [unwired: 3 in, 4 out]
                  n200 = case shown="\"invalid scope\"" w533 {
                    selector: w533 -> [_ w575]
                    tunnel: [w574 w575] -> w532
                    tunnel: w529 -> [w574 _]
                    frame "invalid scope" {
                    }
                    frame Default {
                    }
                  }
                  n201 = Not(x=w536) -> (.not. x?=w535:bool)
                  n202 = Bundle By Name(cluster=w558, "OverrideVIRef"=w547, "NewVIPath"=w538, "ProjectFolder"=w537, "DestroyProjectFolderItem"=w535, "Property"=w519, "PropertyNode"=w518, "Scope"=w532) -> (w557:T8)
                  n203 = Close Reference(reference=w521, error in (no error)=w522) -> ()  [unwired: 1 out]
                  n204 = Close Reference(reference=w541, error in (no error)=w522) -> ()  [unwired: 1 out]
                }
                frame True {
                }
              }
            }
            frame "ReplaceOORefs" {
              n205 = property class="LVClassLibrary"(reference=w602) -> ("Path"=w601:path)  [unwired: 1 in, 2 out]
              n206 = Unbundle By Name(w603) -> ("NewVIPath"=w591:path, "VI"=w594:refnum<vi>)
              n207 = Path To String(path=w601) -> (string=w600:string)
              n208 = call <resource>:"Scripting_SaveVi.vi"("ForceResaving(False)"=TRUE, "error in (no error)"=w597, "NewPath"=w591, "VIRefToSaveIn"=w594) -> ("error out"=w596:errorcluster, "VIRefToSaveOut"=w598:refnum<vi>)  [unwired: 6 in]
              n209 = stacked-sequence {
                tunnel: w596 -> [w607]
                tunnel: [w607] -> w595
                frame #0 {
                  n210 = Wait (ms)(milliseconds to wait=u32 200) -> ()  [unwired: 1 out]
                }
              }
              n211 = call <resource>:"Scripting_ReplaceOORef.vi"("ViRef"=w598, "NewLvClassFile(ProjectPath or LvClassPath)"=w600, "error in (no error)"=w595, "KeepItemsMatchingThisLabel"="(KEEP)$") -> ("error out"=w599:errorcluster)  [unwired: 15 in]
            }
            frame "ReplaceSubVIs" {
              w628 = refnum<vi> refnum  # LVClassLibrary
              # "Get the template Sub VIs and get The\nCurrent SubVIs, replace where the fiile\nname is the same.\n\nIf inheritance, in both this class and the \ntemplate class used, then:\n-Get all SibVIs for the templates base class.\n-Get all SubVIs for this class base class.\n-ANd do the replace of these files in this\nmethod vi, since a sub class method template could\nuse public and protected VIs from the Base Class."
              n212 = Unbundle By Name(w632) -> ("VI"=w618:refnum<vi>, "TemplateName"=w619:string, "Library"=w629:refnum<vi>)
              n213 = property class="LVClassLibrary"(reference=w631, error in=w611) -> (reference out=w630:refnum<vi>, error out=w610:errorcluster, "Path"=w634:path, "Name"=w620:string)
              n214 = Strip Path(path=w634) -> (stripped path=w633:path)  [unwired: 1 out]
              n215 = call-dynamic "GetTemplatePath.vi"("reference in"=w622, "ClassTemplateSubDirectory"=w619, "error in (no error)"=w610) -> ("reference out"=w621:refnum<class "ClassWriterNative.lvclass">, "FolderPathOut"=w638:path, "error out"=w635:errorcluster)  [unwired: 12 in, 2 out]
              n216 = To More Specific Class(target class=w628, reference=w629) -> (specific class reference=w627:refnum<vi>)  [unwired: 1 in, 1 out]
              n217 = call <resource>:"GOOP300_FindFilesToExchange.vi"("OldClassName(Prefix or suffix for some VIs)"=w619, "OldFolderPath"=w638, "NewFolderPath"=w633, "NewClassName(Prefix or suffix for some VIs)"=w620) -> ("OldFiles"=w637:path[], "NewFileArray"=w636:path[])  [unwired: 14 in]
              n218 = call <resource>:"Scripting_ReplaceVisAndControls.vi"("ViRef"=w618, "OldVIsAndControls"=w637, "NewVIsAndControls"=w636, "error in (no error)"=w635) -> ("error out"=w609:errorcluster)  [unwired: 14 in, 1 out]
              n219 = property class="LVClassLibrary"(reference=w627, error in=w609) -> (error out=w608:errorcluster, "Parent"=w617:refnum<vi>)  [unwired: 1 out]
              n220 = property class="LVClassLibrary"(reference=w630, error in=w608) -> ("Parent"=w616:refnum<vi>)  [unwired: 2 out]
              n221 = property class="LVClassLibrary"(reference=w616) -> ("Name"=w614:string)  [unwired: 1 in, 2 out]
              n222 = property class="LVClassLibrary"(reference=w617) -> ("Name"=w615:string)  [unwired: 1 in, 2 out]
              n223 = Equal?(x=w615, y=w614) -> (x = y?=w613:bool)
              n224 = Not A Number/Path/Refnum?(number/path/refnum=w617) -> (NaN/Path/Refnum?=w626:bool)
              n225 = Not A Number/Path/Refnum?(number/path/refnum=w616) -> (NaN/Path/Refnum?=w625:bool)
              n226 = Compound Arithmetic op=OR(w626, w625, w613) -> (w624:bool)
              n227 = case shown="False" w624 {
                tunnel: w609 -> [w657 w661]
                tunnel: [w639 w661] -> w623
                tunnel: w617 -> [w658 w660]
                tunnel: w616 -> [w652 w659]
                tunnel: w618 -> [w644 _]
                tunnel: w621 -> [w650 _]
                frame False {
                  n228 = call <resource>:"GDSLvClass_ReadClassType.vi"("Class Refnum In"=w658, "error in (no error)"=w657) -> ("Class Refnum Out"=w640:refnum<vi>, "ClassSettings"=w651:T29, "error out"=w653:errorcluster)  [unwired: 15 in]
                  n229 = Unbundle By Name(w651) -> ("ClassTemplateUsed"=w642:string)
                  n230 = call <resource>:"GOOP_ClassTemplateSplit.vi"("ClassItemRefIn"=w640, "FullClassTemplate"=w642) -> ("StandardTemplate"=w641:string)  [unwired: 12 in, 1 out]
                  n231 = property class="LVClassLibrary"(reference=w652) -> (reference out=w648:refnum<vi>, error out=w649:errorcluster, "Path"=w647:path, "Name"=w645:string)  [unwired: 1 in]
                  n232 = call-dynamic "GetTemplatePath.vi"("reference in"=w650, "ClassTemplateSubDirectory"=w641, "error in (no error)"=w653) -> ("FolderPathOut"=w654:path, "error out"=w643:errorcluster)  [unwired: 12 in, 3 out]
                  n233 = Strip Path(path=w647) -> (stripped path=w646:path)  [unwired: 1 out]
                  n234 = Close Reference(reference=w648, error in (no error)=w649) -> ()  [unwired: 1 out]
                  n235 = call <resource>:"GOOP300_FindFilesToExchange.vi"("OldClassName(Prefix or suffix for some VIs)"=w641, "OldFolderPath"=w654, "NewFolderPath"=w646, "NewClassName(Prefix or suffix for some VIs)"=w645) -> ("OldFiles"=w655:path[], "NewFileArray"=w656:path[])  [unwired: 14 in]
                  n236 = call <resource>:"Scripting_ReplaceVisAndControls.vi"("ViRef"=w644, "OldVIsAndControls"=w655, "NewVIsAndControls"=w656, "error in (no error)"=w643) -> ("error out"=w639:errorcluster)  [unwired: 14 in, 1 out]
                  n237 = Close Reference(reference=w640, error in (no error)=w639) -> ()  [unwired: 1 out]
                }
                frame True {
                  n238 = Close Reference(reference=w659) -> ()  [unwired: 1 in, 1 out]
                  n239 = Close Reference(reference=w660) -> ()  [unwired: 1 in, 1 out]
                }
              }
            }
            frame "AddViToProject" {
              (unwired) GOOP300_MethodScopeType."Use Parent Folder Scope" ("Scope/Visibility")
              n240 = Unbundle By Name(w685) -> ("PropertyFolderName"=w663:string, "Property"=w664:string, "PropertyNode"=w665:bool, "ProjectFolder"=w691:refnum<vi>, "NewVIPath"=w688:path, "VI"=w682:refnum<vi>, "Scope"=w684:T16)
              n241 = call <resource>:"Scripting_SaveVi.vi"("ForceResaving(False)"=TRUE, "error in (no error)"=w683, "VIRefToSaveIn"=w682) -> ("error out"=w681:errorcluster)  [unwired: 7 in, 1 out]
              n242 = stacked-sequence {
                tunnel: w681 -> [w700]
                tunnel: [w700] -> w680
                frame #0 {
                  n243 = Wait (ms)(milliseconds to wait=u32 5) -> ()  [unwired: 1 out]
                }
              }
              n244 = call <resource>:"AddViToProject.vi"("PropertyFolderName"=w663, "ClassRef"=w662, "Property"=w664, "error out 2"=w680, "PropertyNode"=w665, "NewVIPath"=w688, "ProjectFolder"=w691) -> ("error out"=w667:errorcluster, "AddFile"=w673:refnum<vi>)  [unwired: 3 in]
              n245 = call <resource>:"CommonVIs_Wait.vi"("error in"=w667) -> ("error out"=w666:errorcluster)  [unwired: 9 in]
              n246 = invoke class="LVClassLibrary" method="Set Source Scope"(reference=w662, error in=w666, "SourceRef"=w673, "Scope"=w684) -> (reference out=w670:refnum<vi>, error out=w676:errorcluster)  [unwired: 1 in, 3 out]
              n247 = invoke class="LVClassLibrary" method="Set MustCallParent?"(reference=w670, error in=w676, "DynMemberVI"=w673, "MustOverride"=w671) -> (reference out=w675:refnum<vi>, error out=w674:errorcluster)  [unwired: 1 in, 3 out]
              n248 = Format Into String(format string="Path error:\n%s", w688) -> (resulting string=w679:string)  [unwired: 2 in, 1 out]
              n249 = Bundle By Name(cluster=w685, "ViProjectItem"=w673) -> (w686:T8)
              n250 = invoke class="LVClassLibrary" method="Set MustOverride?"(reference=w675, error in=w674, "DynMemberVI"=w673, "MustOverride"=w672) -> (reference out=w669:refnum<vi>)  [unwired: 1 in, 4 out]
              n251 = invoke class="LVClassLibrary" method="Save"(reference=w669, error in=w666) -> (error out=w678:errorcluster)  [unwired: 2 in, 3 out]
              n252 = case shown="No Error" w678 {
                selector: w678 -> [w693 w698]
                tunnel: w679 -> [_ w696]
                tunnel: [w693 w694] -> w677
                frame No Error {
                  n253 = Wait (ms)(milliseconds to wait=u32 5) -> ()  [unwired: 1 out]
                }
                frame Error {
                  n254 = call <resource>:"GDSError_SetError.vi"("status"=TRUE, "source"=w696) -> ("error out"=w697:errorcluster)  [unwired: 17 in]
                  n255 = call <resource>:"GDSError_MergeError.vi"("error in 1"=w698, "error in 2"=w697) -> ("error out"=w694:errorcluster)  [unwired: 16 in, 1 out]
                }
              }
            }
            frame "CheckDynamicDispatch" {
              (unwired) enum8{"False", "True", "Mixed"}."False" ("TemplateSettings.DynamicDispatch")
              n256 = Unbundle By Name(w708) -> ("TemplateSettings.DynamicDispatch"=w714:enum8{"False", "True", "Mixed"}, "MethodType"=w716:T12)
              n257 = Unbundle By Name(w708) -> ("PropertyNode"=w707:bool)
              n258 = Unbundle By Name(w708) -> ("Property"=w701:string, "VI"=w710:refnum<vi>, "ViProjectItem"=w724:refnum<vi>)
              n259 = invoke class="LVClassLibrary" method="Get Source Scope"(reference=w729, error in=w728, "SourceRef"=w724) -> (error out=w726:errorcluster, "GetSourceScope"=w723:T16)  [unwired: 2 in, 3 out]
              n260 = Equal?(x=w716, y=T12."Override" ("MethodType")) -> (x = y?=w720:bool)
              n261 = Equal?(x=w723, y=T20."private") -> (x = y?=w721:bool)
              n262 = Close Reference(reference=w724, error in (no error)=w726) -> (error out=w725:errorcluster)
              n263 = Compound Arithmetic op=OR(w720, w705) -> (w713:bool)
              n264 = case shown="\"Mixed\"" w714 {
                tunnel: w713 -> [_ _ w780]
                tunnel: [_ TRUE w780] -> w712
                frame "False", Default {
                }
                frame "True" {
                }
                frame "Mixed" {
                }
              }
              n265 = Match Pattern(string=w701, regular expression="^ClassAttribute" ("Left Cell String(Main name)")) -> (offset past match=w703:i32)  [unwired: 1 in, 3 out]
              n266 = Not(x=w721) -> (.not. x?=w715:bool)
              n267 = Greater Or Equal To 0?(x=w703) -> (x >= 0?=w704:bool)
              n268 = Compound Arithmetic op=AND(w707, invert w705) -> (w706:bool)
              n269 = And(x=w715, y=w712) -> (x .and. y?=w719:bool)
              n270 = case shown="False" w711 {
                tunnel: w725 -> [w736 w778]
                tunnel: w719 -> [w732 _]
                tunnel: w716 -> [w735 _]
                tunnel: w710 -> [w734 w777]
                tunnel: [w731 w776] -> w709
                tunnel: w706 -> [w733 _]
                tunnel: w704 -> [w730 _]
                frame False {
                  n271 = case shown="Default" w735 {
                    tunnel: w734 -> [_ w770]
                    tunnel: w736 -> [w746 w769]
                    tunnel: w732 -> [_ w768]
                    tunnel: [w746 w751] -> w731
                    tunnel: w730 -> [_ w747]
                    frame "Af-Method" {
                    }
                    frame Default {
                      # "Set dynamic\ndispatch"
                      n272 = property class="VI"(reference=w770, error in=w769) -> (error out=w751:errorcluster, "ConPane"=w760:refnum<vi>)  [unwired: 1 out]
                      n273 = property class="ConPane" props=["NumConns", "TermBnds[]"](reference=w760, error in=w751) -> (reference out=w759:refnum<vi>, error out=w758:errorcluster, "TermBnds[]"=w755:T31[])  [unwired: 1 out]
                      n274 = for {
                        tunnel: w755 -> [w775] mode=indexing
                        tunnel: [w774] -> w757 mode=indexing
                        tunnel: [w771] -> w756 mode=indexing
                        n275 = Unbundle(w775) -> ("Left"=w773:i16, "Top"=w772:i16)  [unwired: 2 out]
                        n276 = Subtract(x=w773, y=w772) -> (x-y=w771:i16)
                        n277 = Add(x=w773, y=w772) -> (x+y=w774:i16)
                      }
                      n278 = Select(t=T22."Recommended" ("Rule"), s=w747, f=T22."Required" ("Rule")) -> (s? t:f=w748:T22)
                      n279 = Select(t=T22."Dynamic Dispatch" ("Rule"), s=w768, f=w748) -> (s? t:f=w766:T22)
                      n280 = Array Max & Min(array=w756) -> (max index (indices)=w753:i32)  [unwired: 3 out]
                      n281 = Array Max & Min(array=w757) -> (min index (indices)=w754:i32)  [unwired: 3 out]
                      n282 = invoke class="ConPane" method="SetWireRule"(reference=w759, error in=w758, "TermIdx"=w754, "Rule"=w766) -> (reference out=w762:refnum<vi>, error out=w761:errorcluster)  [unwired: 1 in, 3 out]
                      n283 = Select(t=T22."Dynamic Dispatch" ("Rule"), s=w768, f=T22."Recommended" ("Rule")) -> (s? t:f=w763:T22)
                      n284 = invoke class="ConPane" method="SetWireRule"(reference=w762, error in=w761, "TermIdx"=w753, "Rule"=w763) -> (reference out=w752:refnum<vi>)  [unwired: 1 in, 4 out]
                      n285 = Close Reference(reference=w752) -> ()  [unwired: 1 in, 1 out]
                    }
                  }
                  n286 = case shown="True" w733 {
                    tunnel: w734 -> [_ w739]
                    tunnel: [_ w738] -> _
                    tunnel: w731 -> [_ _]
                    frame False {
                    }
                    frame True {
                      n287 = for {
                        N: 3 -> [_]
                        tunnel: w739 -> [w745]
                        tunnel: [w740] -> w738
                        stop <- w740 continue-if-true
                        w742 = TRUE ("Execution:Is Reentrant")
                        n288 = property class="VI"(reference=w745, "Exec.AllowDebug"=FALSE ("Execution:Allow Debugging"), "Exec.ReentrancyType"=T21."Preallocate clone for each instance" ("Execution:Reentrancy Type"), "Exec.IsReentrant"=w742, "ExecInlining"=w742, "Def Err Handling"=FALSE ("Execution:Allow Debugging")) -> (error out=w740:errorcluster)  [unwired: 1 in, 1 out]
                      }
                    }
                  }
                }
                frame True {
                  n289 = call <resource>:"CommonVIs_SetVimProperties.vi"("error in (no error)"=w778, "VIRefIn"=w777) -> ("error out"=w776:errorcluster)  [unwired: 8 in, 1 out]
                }
              }
              n290 = stacked-sequence {
                tunnel: w709 -> [_]
                frame #0 {
                  n291 = Wait (ms)(milliseconds to wait=u32 5) -> ()  [unwired: 1 out]
                }
              }
            }
            frame "UpdateIcon" {
              n292 = property class="LVClassLibrary"(reference=w817, error in=w816) -> (reference out=w786:refnum<vi>, error out=w785:errorcluster, "Is Interface"=w787:bool, "Name"=w804:string)
              n293 = case shown="False" w787 {
                tunnel: w786 -> [w826 w830]
                tunnel: w785 -> [_ w829]
                tunnel: [w821 w828] -> w784
                tunnel: [w822 w827] -> w783
                frame False {
                  n294 = property class="LVClassLibrary"(reference=w826) -> (reference out=w820:refnum<vi>, error out=w825:errorcluster, "Member Data"=w824:refnum<vi>)  [unwired: 1 in]
                  n295 = call <resource>:"GDSLvIcon_AnalyseViIcon(ClassFix).vi"("Class Ref"=w820, "Class Private Data Control VI Ref"=w824, "error in (no error)"=w825) -> ("HeaderIcon"=w821:u8[][], "error out"=w823:errorcluster)  [unwired: 3 in, 12 out]
                  n296 = Close Reference(reference=w824, error in (no error)=w823) -> (error out=w822:errorcluster)
                }
                frame True {
                  n297 = call <resource>:"GDSLvIcon_AnalyseViIcon.vi"("ViRef/LvCLassRef/LvLibRef/ViPath/2D_Image"=w830, "error in (no error)"=w829) -> ("HeaderIcon"=w828:u8[][], "error out"=w827:errorcluster)  [unwired: 4 in, 12 out]
                }
              }
              n298 = Empty Array?(array=w807) -> (empty?=w808:bool)
              n299 = Unbundle By Name(w788) -> ("IconSize"=w790:T4, "ImageRows(32)"=w789:i32)
              n300 = call <resource>:"GDSLvClass_ReadClassColors.vi"("Library Refnum"=w786, "error in (no error)"=w783) -> ("LvClassIconSettings"=w797:T32, "error out"=w805:errorcluster)  [unwired: 12 in, 4 out]
              n301 = Unbundle By Name(w797) -> ("Frame"=w792:u32, "Body Text"=w793:u32, "Frame thickness"=w798:u8)
              n302 = Unbundle By Name(w797) -> ("ColorPublic"=w796:u32, "ColorProtected"=w795:u32, "ColorPrivate"=w794:u32)
              n303 = Unbundle By Name(w819) -> ("Scope"=w802:T16, "VI"=w809:refnum<vi>)
              n304 = case shown="\"protected\"" w802 {
                tunnel: [w832 w833 w834 w835] -> w801
                tunnel: w796 -> [w832 w833 _ _]
                tunnel: w794 -> [_ _ w834 _]
                tunnel: w795 -> [_ _ _ w835]
                frame "invalid scope", Default {
                }
                frame "public" {
                }
                frame "private" {
                }
                frame "protected" {
                }
              }
              n305 = case shown="False" w808 {
                tunnel: w807 -> [w836 _]
                tunnel: [w836 w864] -> w806
                tunnel: w782 -> [_ w862]
                tunnel: w804 -> [_ w860]
                tunnel: w784 -> [_ w851]
                tunnel: w798 -> [_ w850]
                tunnel: w803 -> [_ w848]
                tunnel: w793 -> [_ w847]
                tunnel: w796 -> [_ w846]
                tunnel: w795 -> [_ w844]
                tunnel: w794 -> [_ w843]
                tunnel: w801 -> [_ w842]
                tunnel: w788 -> [_ w841]
                frame False {
                }
                frame True {
                  w853 = u8 32 ("x")
                  n306 = Match Pattern(string=w860, regular expression="\\2e[Ll][Vv][Cc][Ll][Aa][Ss][Ss]") -> (before substring=w859:string)  [unwired: 1 in, 3 out]
                  n307 = Unbundle By Name(w841) -> ("ConnectorPaneHeight"=w839:i32[], "IconSize"=w840:T4)
                  n308 = Array Size(array=w851) -> (size(s)=w858:i32[])
                  n309 = Concatenate Strings(w859, "[_ ]+" ("string")) -> (w868:string)
                  n310 = xnode "Match Regular Expression"("input string"=w862, "regular expression"=w868, "ignore case? (F)"=TRUE) -> ("before match"=w869:string, "after match"=w870:string)  [unwired: 3 in, 3 out]
                  n311 = Multiply(x=w850, y=u8 2) -> (x*y=w855:u8)
                  n312 = Index Array(array=w858) -> (element #1=w856:i32)  [unwired: 2 in, 1 out]
                  n313 = Concatenate Strings(w869, w870) -> (w863:string)
                  n314 = Add(x=w856, y=w855) -> (x+y=w854:i32)
                  n315 = Increment(x=w854) -> (x+1=w852:i32)
                  n316 = Bundle By Name(cluster=T24 {"Text"="", "Allow Only Capital Chars"=TRUE, "Compression"=enum."Auto", "Alignment"=enum."Center"} ("Text"), "Text"=w863) -> (w865:T24)
                  n317 = Subtract(x=w853, y=w852) -> (x-y=w837:i32)
                  n318 = case shown="Default" w840 {
                    selector: w840 -> [_ w875]
                    tunnel: [w872 w873] -> w838
                    tunnel: w839 -> [_ w876]
                    tunnel: w837 -> [w872 _]
                    frame "Full" {
                      (unwired) 32 ("ImageRows(32)")
                    }
                    frame Default {
                      n319 = Array Subset(array=w876, length=w875) -> (w874:i32[])  [unwired: 1 in]
                      n320 = Add Array Elements(numeric array=w874) -> (sum=w873:i32)
                    }
                  }
                  n321 = Subtract(x=w853, y=w855) -> (x-y=w849:u8)
                  n322 = case shown="\"Private\"" w848 {
                    tunnel: w846 -> [_ _ _ w880]
                    tunnel: [w877 w878 w879 w880] -> w845
                    tunnel: w844 -> [_ w878 _ _]
                    tunnel: w843 -> [_ _ w879 _]
                    tunnel: w842 -> [w877 _ _ _]
                    frame "Use Parent Folder Scope", Default {
                    }
                    frame "Protected" {
                    }
                    frame "Private" {
                    }
                    frame "Public" {
                    }
                  }
                  n323 = call <resource>:"GDSLvIcon_GenerateIconText.vi"("Text"=w865, "TextPixelHeight(5-30)"=w838, "Foreground color"=w847, "Background color"=w845, "Text Pixel width(32-FrameThicknes*2))"=w849) -> ("TextOut"=w864:u8[][])  [unwired: 10 in, 4 out]
                }
              }
              n324 = case shown="Default" w790 {
                tunnel: w784 -> [w831 _]
                tunnel: [w831 _] -> w791
                frame Default {
                }
                frame "1 c-term high" {
                }
              }
              n325 = call <resource>:"GDSLvIcon_CreateIconPicture.vi"("FrameColor"=w792, "FrameThickness(1)"=w798, "HeaderIconIn"=w791, "BodyIconIn"=w806, "error in (no error)"=w805, "ImageRows(32)"=w789) -> ("WholeIconOut"=w814:u8[][], "error out"=w811:errorcluster)  [unwired: 8 in, 4 out]
              n326 = Reshape Array(w814, 1024 ("dimension size")) -> (w812:u8[])
              n327 = Bundle By Name(cluster=T23 {"image type"=0, "image depth"=8, "image"=[], "mask"=[], "colors"=[], "Rectangle"={"left"=0, "top"=0, "right"=32, "bottom"=32}} ("image data"), "image"=w812) -> (w810:T23)
              n328 = invoke class="VI" method="VI Icon.Set from Image Data"(reference=w809, error in=w811, "ImageData"=w810) -> (error out=w800:errorcluster)  [unwired: 3 in, 5 out]
            }
            frame "UpdateDescription" {
              n329 = Unbundle By Name(w1006) -> ("App"=w993:refnum<vi>, "VI"=w1009:refnum<vi>, "PropertyNode"=w992:bool)
              n330 = property class="VI"(reference=w1009, error in=w1007, "Description"=w1008) -> (reference out=w1002:refnum<vi>, error out=w999:errorcluster)
              n331 = property class="LVClassLibrary"(reference=w1000, error in=w999) -> (reference out=w998:refnum<vi>, error out=w997:errorcluster, "Name"=w996:string)
              n332 = call <resource>:"GDSLvClass_ReadClassType.vi"("Class Refnum In"=w998, "error in (no error)"=w997) -> ("ClassSettings"=w1004:T29, "error out"=w1003:errorcluster)  [unwired: 15 in, 1 out]
              n333 = Unbundle By Name(w1004) -> ("ConnectorPanePattern"=w995:string)
              n334 = case shown="False" w992 {
                tunnel: w1003 -> [w1015 w1025]
                tunnel: w1002 -> [w1014 _]
                tunnel: [w1013 w1025] -> w1001
                tunnel: w996 -> [w1012 _]
                tunnel: w995 -> [w1010 _]
                tunnel: w993 -> [w1011 _]
                frame False {
                  n335 = case shown="Default" w1010 {
                    tunnel: w1010 -> [_ w1024]
                    tunnel: w1015 -> [w1016 w1022]
                    tunnel: w1014 -> [_ w1021]
                    tunnel: [w1016 w1020] -> w1013
                    tunnel: w1012 -> [_ w1018]
                    tunnel: w1011 -> [_ w1017]
                    frame "" {
                    }
                    frame Default {
                      w1023 = T33 2 items=["4x4x4", "5x6x5", "6x8x6"] ("Pattern")
                      n336 = Scan From String(input string=w1024, default 1=w1023) -> (output 1=w1019:T33)  [unwired: 3 in, 3 out]
                      n337 = call <resource>:"Scripting_SetConnectorPanePattern.vi"("VIPath(s)/ViRef(s)"=w1021, "Pattern"=w1019, "UpdateCallersInThisClassOnly"=w1018, "error in (no error)"=w1022, "AppRef"=w1017) -> ("error out"=w1020:errorcluster)  [unwired: 14 in]
                    }
                  }
                }
                frame True {
                }
              }
            }
            frame "ChangeConnectorPaneLayoutToMatchNewIconSize" {
              n338 = Unbundle By Name(w1031) -> ("IconSize"=w1030:T4)  [unwired: 2 out]
              n339 = Unbundle By Name(w1027) -> ("VI"=w1026:refnum<vi>)
              n340 = case shown="\"Full\", Default" w1030 {
                selector: w1030 -> [_ w1049]
                tunnel: w1029 -> [w1037 w1048]
                tunnel: [w1037 w1039] -> w1028
                tunnel: w1026 -> [_ w1046]
                frame "Full", Default {
                }
                frame "1 c-term high".."3 c-term high" {
                  # "Move any connected controls Up to a free spot.\n1) Get Controls on the removed Connector Pane"
                  n341 = call <resource>:"GOOP_GetControlRearrangement.vi"("VI Refnum"=w1046, "_IconSize"=w1049, "error in (no error)"=w1048, "ShowIconTerminalNumbers"=TRUE) -> ("ControlsToMove"=w1047:T34, "error out"=w1045:errorcluster)  [unwired: 9 in, 5 out]
                  n342 = property class="VI"(reference=w1046, error in=w1045) -> (error out=w1044:errorcluster, "ConPane"=w1040:refnum<vi>)  [unwired: 1 out]
                  n343 = for {
                    tunnel: w1047 -> [w1053] mode=indexing
                    tunnel: w1040 -> [w1055]
                    shift-right: [w1051] -> w1042
                    shift-left: w1044 -> [w1054]
                    tunnel: [w1050] -> w1043 mode=indexing
                    n344 = Unbundle By Name(w1053) -> ("CtrlRef"=w1050:refnum<vi>, "AfterTerminalIndex"=w1052:i32)
                    n345 = invoke class="ConPane" method="AssignCtrlToTerm"(reference=w1055, error in=w1054, "Control"=w1050, "TermIdx"=w1052) -> (error out=w1051:errorcluster)  [unwired: 1 in, 4 out]
                  }
                  n346 = Close Reference(reference=w1043, error in (no error)=w1042) -> (error out=w1041:errorcluster)
                  n347 = Close Reference(reference=w1040, error in (no error)=w1041) -> (error out=w1039:errorcluster)
                }
              }
              n348 = Unbundle By Name(w1027) -> ("DesignPattern"=w1032:bool)
              n349 = Select(t="ApplyDesignPattern", s=w1032, f="ApplyMethodType?") -> (s? t:f=w1033:string)
            }
            frame "ApplyDesignPattern" {
              n350 = Unbundle By Name(w1066) -> ("D-Pattern.ID"=w1063:string, "D-Pattern.Path"=w1064:path, "D-Pattern.Data"=w1060:variant, "VI"=w1058:refnum<vi>, "D-Pattern.Name"=w1056:string)
              n351 = Variant To Data(type=path "", Variant=w1060) -> (data=w1059:path)  [unwired: 1 in, 1 out]
              n352 = Bundle(w1059, "VI"=w1058, "Name"=w1056) -> (w1057:cluster{path, "VI":refnum<vi>, "Name":string})  [unwired: 1 in]
              n353 = Open VI Reference(type specifier VI Refnum (for type only)=refnum<vi> refnum, vi path=w1064, error in (no error)=w1069) -> (vi reference=w1071:refnum<vi>, error out=w1070:errorcluster)  [unwired: 3 in]
              n354 = case shown="No Error" w1070 {
                selector: w1070 -> [w1079 w1083]
                tunnel: w1071 -> [w1082 _]
                tunnel: w1057 -> [w1077 _]
                tunnel: [w1073 w1083] -> w1068
                tunnel: w1067 -> [w1078 _]
                tunnel: w1064 -> [_ _]
                tunnel: w1063 -> [_ _]
                frame No Error {
                  n355 = call-by-ref "?"(reference=w1082, error in=w1079, "Action"=BaseProvider_DesignPatternsActions."CreatePatternMethod", 8:"error in (no error)"=w1079, "DataIn"=w1077, "ClassRefToActOn"=w1078) -> (reference out=w1080:refnum<vi>, error out=w1081:errorcluster, 0:"error out"=w1074:errorcluster)  [unwired: 4 in, 3 out]
                  n356 = Close Reference(reference=w1080, error in (no error)=w1081) -> (error out=w1075:errorcluster)
                  n357 = Merge Errors(w1075, w1074) -> (w1073:errorcluster)
                }
                frame Error {
                }
              }
            }
            frame "ApplyMethodType?" {
              n358 = Unbundle By Name(w1089) -> ("MethodType"=w1094:T12, "VI"=w1092:refnum<vi>)
              n359 = Unbundle By Name(w1089) -> ("Property"=w1091:string, "OverrideVIRef"=w1087:refnum<vi>, "TemplateFolder"=w1084:path)
              n360 = case shown="\"Property\"" w1094 {
                tunnel: w1093 -> [w1096 w1107 w1145]
                tunnel: [w1096 w1103 w1136] -> w1088
                tunnel: w1092 -> [_ w1105 w1137]
                tunnel: w1091 -> [_ w1109 _]
                tunnel: w1090 -> [_ w1101 _]
                tunnel: w1087 -> [_ _ w1155]
                tunnel: w1086 -> [_ w1106 _]
                tunnel: w1085 -> [_ w1108 _]
                tunnel: w1084 -> [_ _ w1144]
                frame "Normal", Default {
                }
                frame "Property" {
                  n361 = disable-structure shown="Enabled" {
                    disable-tunnel: w1105 -> [w1133 w1134]
                    disable-tunnel: [w1132 w1134] -> w1104
                    frame Disabled {
                      n362 = invoke class="VI" method="FP.Open"(reference=w1133) -> (reference out=w1132:refnum<vi>)  [unwired: 4 in, 4 out]
                    }
                    frame Enabled {
                    }
                  }
                  n363 = call <resource>:"GOOP400_ConfigurationMemory.vi"("Action"=enum16{"Read", "Load", "Save"}."Read") -> ("OptionsOut"=w1099:T28)  [unwired: 17 in, 1 out]
                  n364 = Unbundle By Name(w1099) -> ("CleanUpBDForPropertyMethods"=w1097:bool)
                  n365 = property class="LVClassLibrary"(reference=w1101) -> (error out=w1100:errorcluster, "Is Interface"=w1102:bool)  [unwired: 1 in, 1 out]
                  n366 = case shown="False" w1102 {
                    tunnel: w1109 -> [w1118 _]
                    tunnel: w1108 -> [w1117 _]
                    tunnel: w1107 -> [w1116 w1131]
                    tunnel: w1106 -> [w1115 _]
                    tunnel: w1104 -> [w1111 _]
                    tunnel: [w1113 w1131] -> w1103
                    tunnel: w1101 -> [w1112 _]
                    tunnel: w1100 -> [_ _]
                    tunnel: w1097 -> [w1110 _]
                    frame False {
                      n367 = call-dynamic "ApplyPropertyTemplateToMethod.vi"("ClassWriterNative in"=w1117, "VIRef"=w1111, "ClassRef"=w1112, "PropertyName"=w1118, "MethodTemplateName"=w1115, "error in (no error)"=w1116) -> ("error out"=w1114:errorcluster)  [unwired: 12 in, 1 out]
                      n368 = disable-structure shown="Enabled" {
                        disable-tunnel: w1111 -> [w1121 w1122]
                        disable-tunnel: w1114 -> [w1120 w1124]
                        disable-tunnel: [w1119 w1126] -> w1113
                        disable-tunnel: w1110 -> [_ w1125]
                        frame Disabled {
                          n369 = call <resource>:"Scripting_SaveUpdateSubVIs.vi"("error in (no error)"=w1120, "VI Refnum"=w1121) -> ("error out"=w1119:errorcluster)  [unwired: 9 in]
                        }
                        frame Enabled {
                          n370 = call "Scripting_AlignToConnectorPane.vi"("error in (no error)"=w1124, "VI Ref"=w1122) -> ("error out"=w1123:errorcluster)  [unwired: 9 in]
                          n371 = case shown="True" w1125 {
                            tunnel: w1123 -> [w1127 w1130]
                            tunnel: w1122 -> [_ w1129]
                            tunnel: [w1127 w1128] -> w1126
                            frame False {
                            }
                            frame True {
                              n372 = invoke class="VI" method="BD.CleanUp"(reference=w1129, error in=w1130) -> (error out=w1128:errorcluster)  [unwired: 1 in, 2 out]
                            }
                          }
                        }
                      }
                    }
                    frame True {
                    }
                  }
                }
                frame "Override" {
                  w1146 = "OverrideMethodControlsToIgnore" ("section")
                  # "[OverrideMethodControlsToIgnore]\n1=timeout in ms (-1)\n2=time left\n3=timed out?"
                  n373 = Build Path(base path=w1144, name or relative path="methods.ini") -> (appended path=w1152:path)
                  n374 = call <vilib>:"Open Config Data.vi"("error in (no error)"=w1145, "create file if necessary (T)"=FALSE ("create file if necessary? (T)"), "configuration file path"=w1152) -> ("error out"=w1151:errorcluster, "refnum"=w1150:T35)  [unwired: 6 in, 1 out]
                  n375 = call <vilib>:"Get Key Names.vi"("section"=w1146, "error in (no error)"=w1151, "refnum"=w1150) -> ("error out"=w1149:errorcluster, "key names"=w1147:string[], "refnum out"=w1148:T35)  [unwired: 5 in, 1 out]
                  n376 = for {
                    shift-right: [w1165] -> w1143
                    shift-left: w1149 -> [w1172]
                    shift-right: [w1166] -> w1142
                    shift-left: w1148 -> [w1171]
                    tunnel: w1147 -> [w1170] mode=indexing
                    tunnel: w1146 -> [w1168]
                    tunnel: [w1167] -> w1139 mode=indexing
                    n377 = call-poly <vilib>:"Read Key.vi"("read raw string? (F)"=TRUE ("create file if necessary? (T)"), "section"=w1168, "error in (no error)"=w1172, "key"=w1170, "refnum"=w1171) -> ("error out"=w1165:errorcluster, "value"=w1167:string, "refnum out"=w1166:T35)  [unwired: 3 in, 1 out]
                  }
                  n378 = call <vilib>:"Close Config Data.vi"("error in (no error)"=w1143, "write file if changed (T)"=FALSE ("write configuration file? (T)"), "refnum"=w1142) -> ("error out"=w1140:errorcluster)  [unwired: 7 in, 1 out]
                  n379 = Empty Array?(array=w1139) -> (empty?=w1138:bool)
                  n380 = case shown="True" w1138 {
                    tunnel: w1155 -> [w1159 w1164]
                    tunnel: w1140 -> [w1158 w1163]
                    tunnel: w1137 -> [w1157 w1162]
                    tunnel: [w1156 w1161] -> w1135
                    tunnel: w1139 -> [_ w1160]
                    frame True {
                      n381 = call <resource>:"MergeOverrideViWithMethod_V2.vi"("error in"=w1158, "OverrideVIRef"=w1159, "ViRef"=w1157) -> ("error out"=w1156:errorcluster)  [unwired: 8 in]
                    }
                    frame False {
                      n382 = call <resource>:"MergeOverrideViWithMethod.vi"("ViRef"=w1162, "OverrideVIRef"=w1164, "GetControlNamesThatShouldBeIgnored"=w1160, "error in"=w1163) -> ("error out"=w1161:errorcluster)  [unwired: 15 in]
                    }
                  }
                  n383 = call "Scripting_AlignToConnectorPane.vi"("error in (no error)"=w1135, "VI Ref"=w1137) -> ("error out"=w1136:errorcluster)  [unwired: 9 in]
                }
              }
            }
            frame "CloseRefs", "Error", Default {
              n384 = Unbundle By Name(w1182) -> ("SubVIs"=w1177:refnum<vi>[], "DestroyProjectFolderItem"=w1188:bool, "ProjectFolder"=w1192:refnum<vi>, "Library"=w1181:refnum<vi>, "VI"=w1191:refnum<vi>, "App"=w1173:refnum<vi>, "NewVIPath"=w1175:path)
              n385 = case shown="\"CloseRefs\"" w1185 {
                tunnel: w1191 -> [w1202 w1204]
                tunnel: w1190 -> [w1201 w1206]
                tunnel: w1189 -> [_ w1217]
                tunnel: [w1201 w1208] -> w1187
                tunnel: [w1202 w1214] -> w1186
                tunnel: w1176 -> [_ w1212]
                tunnel: w1173 -> [_ w1211]
                tunnel: w1175 -> [_ w1210]
                tunnel: w1174 -> [_ w1207]
                tunnel: w1173 -> [_ w1203]
                frame Default {
                }
                frame "CloseRefs" {
                  n386 = call "Scripting_FixBrokenVI.vi"("AppRef"=w1203, "error in (no error)"=w1206, "ViPath/ViName"=w1204) -> ("error out"=w1205:errorcluster)  [unwired: 8 in]
                  n387 = property class="VI"(reference=w1204, error in=w1205, "Front Panel.Open"=w1217) -> (reference out=w1215:refnum<vi>, error out=w1216:errorcluster)
                  n388 = call <resource>:"Scripting_SaveVi.vi"("ForceResaving(False)"=TRUE, "error in (no error)"=w1216, "VIRefToSaveIn"=w1215) -> ("error out"=w1209:errorcluster, "VIRefToSaveOut"=w1214:refnum<vi>)  [unwired: 7 in]
                  n389 = case shown="True" w1212 {
                    tunnel: w1211 -> [_ w1223]
                    tunnel: w1210 -> [_ w1222]
                    tunnel: w1209 -> [w1218 w1221]
                    tunnel: [w1218 w1220] -> w1208
                    tunnel: w1207 -> [_ w1219]
                    frame False {
                    }
                    frame True {
                      n390 = call <resource>:"MM.vi"("AppInst"=w1223, "ActorMethod"=w1222, "ActorClassItemRef(Don't Delete)"=w1219, "error in"=w1221) -> ("error out"=w1220:errorcluster)  [unwired: 15 in]
                    }
                  }
                }
              }
              n391 = Close Reference(reference=w1186, error in (no error)=w1187) -> (error out=w1194:errorcluster)
              n392 = Not A Number/Path/Refnum?(number/path/refnum=w1181) -> (NaN/Path/Refnum?=w1180:bool)
              n393 = case shown="False" w1180 {
                tunnel: w1194 -> [w1199 w1200]
                tunnel: [w1198 w1200] -> w1193
                tunnel: w1181 -> [w1197 _]
                frame False {
                  n394 = Close Reference(reference=w1197, error in (no error)=w1199) -> (error out=w1198:errorcluster)
                }
                frame True {
                }
              }
              n395 = case shown="True" w1188 {
                tunnel: w1193 -> [w1224 w1227]
                tunnel: w1192 -> [_ w1226]
                tunnel: [w1224 w1225] -> w1178
                frame False {
                }
                frame True {
                  n396 = Close Reference(reference=w1226, error in (no error)=w1227) -> (error out=w1225:errorcluster)
                }
              }
              n397 = Close Reference(reference=w1177, error in (no error)=w1178) -> ()  [unwired: 1 out]
              n398 = Close Reference(reference=w1173, error in (no error)=w1178) -> (error out=w1179:errorcluster)
              n399 = call <resource>:"GDSError_LogErrorInformation.vi"("State"=w1183, "LocalVariableData"=w1182, "error in (no error)"=w1179) -> ("error out"=w1184:errorcluster)  [unwired: 16 in]
            }
          }
          n400 = Equal?(x=w168, y="Exit") -> (x = y?=w172:bool)
          n401 = Select(t="Error", s=w165, f=w168) -> (s? t:f=w171:string)
        }
        n402 = Unbundle By Name(w122) -> ("NewVIPath"=w121:path)
      }
    }
    frame Error {
    }
  }
  "ClassWriterNative.lvclass 2" <- w20
  "error out" <- w22
  "MethodPaths" <- w1
  "ClassItemRefOut" <- "ClassItemRefIn"
